vi "符合分析1.7.vi"(5 "大于信号周期":dbl, 6 "length":dbl=200.0 format="%#_13g", 7 "小于信号周期":dbl=500000.0, 8 "min bin":i32=100, 9 "通道B":i32=12, 10 "通道A":i32=1, 11 "file path (dialog if empty)":path=path "G:/tdc/2017/data/test_20250731_124932.csv") -> (0 "standard deviation[ps]":dbl=0.476370061755716 format="%0.2f", 1 "Fitting Sigma":dbl=0.8923286870726619, 2 "Fitting center":dbl=0.5, 3 "mean[ps]":dbl=-0.34797707935405453 format="%0.2f")   [LabVIEW 2017]
uses:
  <vilib>/Utility/file.llb/Read Delimited Spreadsheet (DBL).vi
  <vilib>/Analysis/NI_AALBase.lvlib
panel:
  out "Numeric 2":dbl=110111087360.0 format="%#_16f"
  out "Numeric":dbl=110111087360.0 format="%#_16f"
  out "求和":dbl
  out "x/y":dbl=nan
  out "已经读取的行数":i32=40006
  in  "type (empty)":dbl[][](array[numeric]) caption="类型（空）" format="%0.2f"
  out "错误输出":errorcluster={"status"=TRUE, "code"=4, "source"="Read from Text File in 符合分析1.7.vi<APPEND>\nG:\\tdc\\2017\\data\\test_20250731_124932.csv"}
  in  "单词循环读取的行数":i32=20003
  out "mean[ps] 3":dbl=-185.2719139547909 format="%0.2f"
  out "mean[ps] 2":dbl=-343.16432726517195 format="%0.2f"
  in  "single board":bool=TRUE
  out "offset1":dbl
  out "size(s) 3":i32=64
  in  "calib":bool
  out "offset0":dbl
  in  "file path (dialog if empty) 2":path=path "D:/labview/diff.csv"
  out "数值":i32=2110
  out "大小":i32
  out "Histogram 2":dynamicdata(graph)=[{"t0"=timestamp(500000 s since 1904-01-01), "dt"=1000000.0, "Y"=array[1000 elements], "attributes"=variant("NI_ChannelName"=variant(string " (Histogram)"), "NI_ExpIsRelativeTime"=variant(bool TRUE), "NI_ExpStartTimeStamp"=variant(timestamp timestamp(3836782584.3645935 s since 1904-01-01)), "NI_ExpTimeStamp"=variant(timestamp timestamp(3836782584.3645935 s since 1904-01-01)), "NI_ExpXDimension"=variant(string "BIN"), "NI_OriginalChannelName"=variant(string ""))}] caption="直方图"
  in  "禁用的索引 (列)":i32=6
  in  "window":dbl=200.0 format="%#_13g"
  in  "intervals":i32=1000
  in  "min":dbl=-500.0 format="%#_13g"
  in  "max":dbl=500.0 format="%#_13g"
  out "XY Graph":cluster{"X":dbl, "Y":dbl}[](graph)=[{"X"=107773084761.0, "Y"=0.0}, {"X"=107774084760.0, "Y"=-1.0}, {"X"=107775084760.0, "Y"=0.0}, {"X"=107778084768.0, "Y"=-1.0}, {"X"=107779084768.0, "Y"=0.0}, {"X"=107782084777.0, "Y"=0.0}, {"X"=107793084792.0, "Y"=0.0}, {"X"=107805084816.0, "Y"=-1.0}, {"X"=107809084825.0, "Y"=0.0}, {"X"=107810084824.0, "Y"=-1.0}, {"X"=107814084832.0, "Y"=-1.0}, {"X"=107818084841.0, "Y"=0.0}, {"X"=107827084857.0, "Y"=0.0}, {"X"=107829084856.0, "Y"=0.0}, {"X"=107832084864.0, "Y"=-1.0}, {"X"=107833084864.0, "Y"=0.0}, {"X"=107836084873.0, "Y"=0.0}, {"X"=107837084872.0, "Y"=-1.0}, {"X"=107841084880.0, "Y"=-1.0}, {"X"=107851084896.0, "Y"=0.0}, {"X"=107856084840.0, "Y"=0.0}, {"X"=107859084848.0, "Y"=-1.0}, {"X"=107860084848.0, "Y"=0.0}, {"X"=107863084857.0, "Y"=0.0}, {"X"=107868084864.0, "Y"=-1.0}, {"X"=107872084873.0, "Y"=0.0}, {"X"=107873084872.0, "Y"=-1.0}, {"X"=107878084880.0, "Y"=0.0}, {"X"=107883084888.0, "Y"=0.0}, {"X"=107887084896.0, "Y"=0.0}, {"X"=107891084904.0, "Y"=-1.0}, {"X"=107892084904.0, "Y"=0.0}, {"X"=107895084912.0, "Y"=-1.0}, {"X"=107896084912.0, "Y"=0.0}, {"X"=107899084921.0, "Y"=0.0}, {"X"=107900084920.0, "Y"=-1.0}, {"X"=107901084920.0, "Y"=0.0}, {"X"=107910084904.0, "Y"=0.0}, {"X"=107914084912.0, "Y"=0.0}, {"X"=107915084912.0, "Y"=0.0}, {"X"=107919084920.0, "Y"=0.0}, {"X"=107926084937.0, "Y"=0.0}, {"X"=107935084953.0, "Y"=0.0}, {"X"=107941084960.0, "Y"=0.0}, {"X"=107944084969.0, "Y"=0.0}, {"X"=107950084976.0, "Y"=0.0}, {"X"=107951084976.0, "Y"=0.0}, {"X"=107954084984.0, "Y"=-1.0}, {"X"=107958084993.0, "Y"=0.0}, {"X"=107960084992.0, "Y"=0.0}, {"X"=107963085000.0, "Y"=-1.0}, {"X"=107969085008.0, "Y"=0.0}, {"X"=107973085016.0, "Y"=0.0}, {"X"=107978085024.0, "Y"=0.0}, {"X"=107985085041.0, "Y"=0.0}, {"X"=107994085057.0, "Y"=0.0}, {"X"=108000085064.0, "Y"=0.0}, {"X"=108004085072.0, "Y"=-1.0}, {"X"=108005085072.0, "Y"=0.0}, {"X"=108007085081.0, "Y"=0.0}, {"X"=108008085080.0, "Y"=-1.0}, {"X"=108009085080.0, "Y"=0.0}, {"X"=108012085089.0, "Y"=0.0}, {"X"=108013085088.0, "Y"=-1.0}, {"X"=108014085088.0, "Y"=0.0}, {"X"=108021085105.0, "Y"=0.0}, {"X"=108022085104.0, "Y"=0.0}, {"X"=108023085104.0, "Y"=0.0}, {"X"=108026085112.0, "Y"=-1.0}, {"X"=108027085112.0, "Y"=0.0}, {"X"=108031085120.0, "Y"=-1.0}, {"X"=108032085120.0, "Y"=0.0}, {"X"=108036085128.0, "Y"=0.0}, {"X"=108039085137.0, "Y"=0.0}, {"X"=108041085136.0, "Y"=0.0}, {"X"=108044085144.0, "Y"=-1.0}, {"X"=108048085153.0, "Y"=0.0}, {"X"=108058085168.0, "Y"=-1.0}, {"X"=108059085168.0, "Y"=0.0}, {"X"=108063085176.0, "Y"=0.0}, {"X"=108066085185.0, "Y"=0.0}, {"X"=108067085184.0, "Y"=-1.0}, {"X"=108075085201.0, "Y"=0.0}, {"X"=108080085208.0, "Y"=-1.0}, {"X"=108085085216.0, "Y"=-1.0}, {"X"=108086085216.0, "Y"=0.0}, {"X"=108090085224.0, "Y"=0.0}, {"X"=108094085232.0, "Y"=-1.0}, {"X"=108097085241.0, "Y"=0.0}, {"X"=108116085272.0, "Y"=-1.0}, {"X"=108117085272.0, "Y"=0.0}, {"X"=108121085280.0, "Y"=-1.0}, {"X"=108125085288.0, "Y"=-1.0}, {"X"=108129085297.0, "Y"=0.0}, {"X"=108138085313.0, "Y"=0.0}, {"X"=108143085240.0, "Y"=-1.0}, {"X"=108144085240.0, "Y"=0.0}, {"X"=108148085248.0, "Y"=-1.0}, {"X"=108149085248.0, "Y"=0.0}, {"X"=108153085256.0, "Y"=0.0}, {"X"=108156085265.0, "Y"=0.0}, {"X"=108175085296.0, "Y"=-1.0}, {"X"=108179085304.0, "Y"=-1.0}, {"X"=108187085321.0, "Y"=0.0}, {"X"=108188085320.0, "Y"=-1.0}, {"X"=108197085336.0, "Y"=-1.0}, {"X"=108203085344.0, "Y"=0.0}, {"X"=108207085288.0, "Y"=0.0}, {"X"=108219085313.0, "Y"=0.0}, {"X"=108225085320.0, "Y"=0.0}, {"X"=108233085336.0, "Y"=-1.0}, {"X"=108234085336.0, "Y"=0.0}, {"X"=108238085344.0, "Y"=-1.0}, {"X"=108242085352.0, "Y"=-1.0}, {"X"=108243085352.0, "Y"=0.0}, {"X"=108246085361.0, "Y"=0.0}, {"X"=108247085360.0, "Y"=-1.0}, {"X"=108252085368.0, "Y"=0.0}, {"X"=108256085376.0, "Y"=-1.0}, {"X"=108257085376.0, "Y"=0.0}, {"X"=108261085384.0, "Y"=0.0}, {"X"=108265085392.0, "Y"=-1.0}, {"X"=108266085392.0, "Y"=0.0}, {"X"=108269085400.0, "Y"=-1.0}, {"X"=108273085409.0, "Y"=0.0}, {"X"=108275085408.0, "Y"=0.0}, {"X"=108277085417.0, "Y"=0.0}, {"X"=108284085392.0, "Y"=0.0}, {"X"=108287085400.0, "Y"=-1.0}, {"X"=108292085408.0, "Y"=-1.0}, {"X"=108296085416.0, "Y"=-1.0}, {"X"=108300085425.0, "Y"=0.0}, {"X"=108301085424.0, "Y"=-1.0}, {"X"=108305085432.0, "Y"=-1.0}, {"X"=108306085432.0, "Y"=0.0}, {"X"=108309085441.0, "Y"=0.0}, {"X"=108311085440.0, "Y"=0.0}, {"X"=108314085448.0, "Y"=-1.0}, {"X"=108319085456.0, "Y"=-1.0}, {"X"=108324085464.0, "Y"=0.0}, {"X"=108328085472.0, "Y"=-1.0}, {"X"=108331085481.0, "Y"=0.0}, {"X"=108333085480.0, "Y"=0.0}, {"X"=108336085489.0, "Y"=0.0}, {"X"=108340085497.0, "Y"=0.0}, {"X"=108345085505.0, "Y"=0.0}, {"X"=108350085512.0, "Y"=-1.0}, {"X"=108355085520.0, "Y"=-1.0}, {"X"=108359085528.0, "Y"=-1.0}, {"X"=108367085545.0, "Y"=0.0}, {"X"=108374085552.0, "Y"=0.0}, {"X"=108378085448.0, "Y"=0.0}, {"X"=108386085464.0, "Y"=-1.0}, {"X"=108387085464.0, "Y"=0.0}, {"X"=108390085473.0, "Y"=0.0}, {"X"=108409085504.0, "Y"=-1.0}, {"X"=108417085521.0, "Y"=0.0}, {"X"=108418085520.0, "Y"=0.0}, {"X"=108421085529.0, "Y"=0.0}, {"X"=108436085552.0, "Y"=0.0}, {"X"=108437085552.0, "Y"=0.0}, {"X"=108440085560.0, "Y"=-1.0}, {"X"=108441085560.0, "Y"=0.0}, {"X"=108445085568.0, "Y"=-1.0}, {"X"=108448085577.0, "Y"=0.0}, {"X"=108462085601.0, "Y"=0.0}, {"X"=108464085600.0, "Y"=0.0}, {"X"=108467085608.0, "Y"=-1.0}, {"X"=108468085608.0, "Y"=0.0}, {"X"=108471085617.0, "Y"=0.0}, {"X"=108472085616.0, "Y"=0.0}, {"X"=108475085625.0, "Y"=0.0}, {"X"=108476085624.0, "Y"=-1.0}, {"X"=108480085633.0, "Y"=0.0}, {"X"=108484085641.0, "Y"=0.0}, {"X"=108485085640.0, "Y"=-1.0}, {"X"=108491085648.0, "Y"=0.0}, {"X"=108494085656.0, "Y"=-1.0}, {"X"=108495085656.0, "Y"=0.0}, {"X"=108499085664.0, "Y"=0.0}, {"X"=108500085664.0, "Y"=0.0}, {"X"=108509085680.0, "Y"=0.0}, {"X"=108511085689.0, "Y"=0.0}, {"X"=108518085696.0, "Y"=0.0}, {"X"=108521085704.0, "Y"=-1.0}, {"X"=108530085688.0, "Y"=-1.0}, {"X"=108534085697.0, "Y"=0.0}, {"X"=108538085705.0, "Y"=0.0}, {"X"=108539085704.0, "Y"=-1.0}, {"X"=108543085713.0, "Y"=0.0}, {"X"=108549085720.0, "Y"=0.0}, {"X"=108553085728.0, "Y"=0.0}, {"X"=108554085728.0, "Y"=0.0}, {"X"=108557085736.0, "Y"=-1.0}, {"X"=108558085736.0, "Y"=0.0}, {"X"=108562085744.0, "Y"=0.0}, {"X"=108565085753.0, "Y"=0.0}, {"X"=108581085680.0, "Y"=0.0}, {"X"=108584085688.0, "Y"=-1.0}, {"X"=108592085705.0, "Y"=0.0}, {"X"=108593085704.0, "Y"=-1.0}, {"X"=108597085713.0, "Y"=0.0}, {"X"=108601085721.0, "Y"=0.0}, {"X"=108608085728.0, "Y"=0.0}, {"X"=108612085736.0, "Y"=0.0}, {"X"=108616085744.0, "Y"=0.0}, {"X"=108620085752.0, "Y"=-1.0}, {"X"=108621085752.0, "Y"=0.0}, {"X"=108643085648.0, "Y"=0.0}, {"X"=108647085656.0, "Y"=-1.0}, {"X"=108652085664.0, "Y"=0.0}, {"X"=108655085609.0, "Y"=0.0}, {"X"=108662085616.0, "Y"=0.0}, {"X"=108666085624.0, "Y"=0.0}, {"X"=108670085632.0, "Y"=0.0}, {"X"=108671085632.0, "Y"=0.0}, {"X"=108674085640.0, "Y"=-1.0}, {"X"=108675085640.0, "Y"=0.0}, {"X"=108678085649.0, "Y"=0.0}, {"X"=108680085648.0, "Y"=0.0}, {"X"=108682085657.0, "Y"=0.0}, {"X"=108684085656.0, "Y"=0.0}, {"X"=108689085664.0, "Y"=0.0}, {"X"=108693085672.0, "Y"=0.0}, {"X"=108696085681.0, "Y"=0.0}, {"X"=108698085680.0, "Y"=0.0}, {"X"=108701085688.0, "Y"=-1.0}, {"X"=108705085697.0, "Y"=0.0}, {"X"=108706085696.0, "Y"=0.0}, {"X"=108710085704.0, "Y"=-1.0}, {"X"=108711085704.0, "Y"=0.0}, {"X"=108714085713.0, "Y"=0.0}, {"X"=108716085712.0, "Y"=0.0}, {"X"=108718085721.0, "Y"=0.0}, {"X"=108720085720.0, "Y"=0.0}, {"X"=108725085728.0, "Y"=0.0}, {"X"=108729085736.0, "Y"=0.0}, {"X"=108733085744.0, "Y"=0.0}, {"X"=108737085752.0, "Y"=-1.0}, {"X"=108742085760.0, "Y"=0.0}, {"X"=108752085712.0, "Y"=0.0}, {"X"=108760085728.0, "Y"=-1.0}, {"X"=108764085736.0, "Y"=-1.0}, {"X"=108768085745.0, "Y"=0.0}, {"X"=108769085744.0, "Y"=-1.0}, {"X"=108772085753.0, "Y"=0.0}, {"X"=108773085752.0, "Y"=-1.0}, {"X"=108779085760.0, "Y"=0.0}, {"X"=108783085768.0, "Y"=0.0}, {"X"=108786085777.0, "Y"=0.0}, {"X"=108787085776.0, "Y"=-1.0}, {"X"=108788085776.0, "Y"=0.0}, {"X"=108791085784.0, "Y"=-1.0}, {"X"=108792085784.0, "Y"=0.0}, {"X"=108795085793.0, "Y"=0.0}, {"X"=108796085792.0, "Y"=-1.0}, {"X"=108801085800.0, "Y"=0.0}, {"X"=108815085744.0, "Y"=0.0}, {"X"=108818085752.0, "Y"=-1.0}, {"X"=108822085761.0, "Y"=0.0}, {"X"=108823085760.0, "Y"=-1.0}, {"X"=108827085768.0, "Y"=-1.0}, {"X"=108837085656.0, "Y"=0.0}, {"X"=108842085664.0, "Y"=0.0}, {"X"=108845085672.0, "Y"=-1.0}, {"X"=108854085688.0, "Y"=-1.0}, {"X"=108869085712.0, "Y"=0.0}, {"X"=108873085720.0, "Y"=0.0}, {"X"=108876085729.0, "Y"=0.0}, {"X"=108881085736.0, "Y"=-1.0}, {"X"=108885085745.0, "Y"=0.0}, {"X"=108895085632.0, "Y"=-1.0}, {"X"=108896085632.0, "Y"=0.0}, {"X"=108900085640.0, "Y"=0.0}, {"X"=108904085648.0, "Y"=-1.0}, {"X"=108905085648.0, "Y"=0.0}, {"X"=108908085656.0, "Y"=-1.0}, {"X"=108913085664.0, "Y"=-1.0}, {"X"=108917085672.0, "Y"=-1.0}, {"X"=108923085680.0, "Y"=0.0}, {"X"=108927085688.0, "Y"=0.0}, {"X"=108932085696.0, "Y"=0.0}, {"X"=108935085704.0, "Y"=-1.0}, {"X"=108939085713.0, "Y"=0.0}, {"X"=108944085720.0, "Y"=-1.0}, {"X"=108948085729.0, "Y"=0.0}, {"X"=108954085736.0, "Y"=0.0}, {"X"=108957085745.0, "Y"=0.0}, {"X"=108958085744.0, "Y"=-1.0}, {"X"=108959085744.0, "Y"=0.0}, {"X"=108962085752.0, "Y"=-1.0}, {"X"=108963085752.0, "Y"=0.0}, {"X"=108966085761.0, "Y"=0.0}, {"X"=108967085760.0, "Y"=-1.0}, {"X"=108971085768.0, "Y"=-1.0}, {"X"=108976085776.0, "Y"=-1.0}, {"X"=108981085784.0, "Y"=0.0}, {"X"=108986085792.0, "Y"=0.0}, {"X"=108993085809.0, "Y"=0.0}, {"X"=108994085808.0, "Y"=-1.0}, {"X"=108995085808.0, "Y"=0.0}, {"X"=108998085816.0, "Y"=-1.0}, {"X"=109003085824.0, "Y"=-1.0}, {"X"=109017085848.0, "Y"=0.0}, {"X"=109020085857.0, "Y"=0.0}, {"X"=109021085856.0, "Y"=-1.0}, {"X"=109022085856.0, "Y"=0.0}, {"X"=109025085864.0, "Y"=-1.0}, {"X"=109026085864.0, "Y"=0.0}, {"X"=109029085873.0, "Y"=0.0}, {"X"=109040085888.0, "Y"=0.0}, {"X"=109044085896.0, "Y"=0.0}, {"X"=109045085896.0, "Y"=0.0}, {"X"=109049085904.0, "Y"=0.0}, {"X"=109054085912.0, "Y"=0.0}, {"X"=109056085921.0, "Y"=0.0}, {"X"=109066085936.0, "Y"=-1.0}, {"X"=109071085944.0, "Y"=0.0}, {"X"=109075085952.0, "Y"=-1.0}, {"X"=109076085952.0, "Y"=0.0}, {"X"=109079085960.0, "Y"=-1.0}, {"X"=109083085969.0, "Y"=0.0}, {"X"=109084085968.0, "Y"=-1.0}, {"X"=109088085976.0, "Y"=-1.0}, {"X"=109098085992.0, "Y"=0.0}, {"X"=109099085992.0, "Y"=0.0}, {"X"=109103086000.0, "Y"=0.0}, {"X"=109107086008.0, "Y"=0.0}, {"X"=109110086017.0, "Y"=0.0}, {"X"=109119086033.0, "Y"=0.0}, {"X"=109129086048.0, "Y"=-1.0}, {"X"=109134086056.0, "Y"=0.0}, {"X"=109137086065.0, "Y"=0.0}, {"X"=109138086064.0, "Y"=-1.0}, {"X"=109142086072.0, "Y"=-1.0}, {"X"=109144086072.0, "Y"=0.0}, {"X"=109146086081.0, "Y"=0.0}, {"X"=109147086080.0, "Y"=-1.0}, {"X"=109157086096.0, "Y"=0.0}, {"X"=109161086104.0, "Y"=0.0}, {"X"=109162086104.0, "Y"=0.0}, {"X"=109166086112.0, "Y"=0.0}, {"X"=109169086120.0, "Y"=-1.0}, {"X"=109171086008.0, "Y"=0.0}, {"X"=109173086017.0, "Y"=0.0}, {"X"=109182086033.0, "Y"=0.0}, {"X"=109188086040.0, "Y"=0.0}, {"X"=109192086048.0, "Y"=-1.0}, {"X"=109193086048.0, "Y"=0.0}, {"X"=109196086056.0, "Y"=-1.0}, {"X"=109200086065.0, "Y"=0.0}, {"X"=109205086072.0, "Y"=-1.0}, {"X"=109207086072.0, "Y"=0.0}, {"X"=109210086080.0, "Y"=-1.0}, {"X"=109215086088.0, "Y"=0.0}, {"X"=109216086088.0, "Y"=0.0}, {"X"=109220086096.0, "Y"=0.0}, {"X"=109224086104.0, "Y"=0.0}, {"X"=109225086104.0, "Y"=0.0}, {"X"=109227086113.0, "Y"=0.0}, {"X"=109229086112.0, "Y"=0.0}, {"X"=109232086120.0, "Y"=-1.0}, {"X"=109234086120.0, "Y"=0.0}, {"X"=109241086136.0, "Y"=-1.0}, {"X"=109243086136.0, "Y"=0.0}, {"X"=109246086144.0, "Y"=-1.0}, {"X"=109247086144.0, "Y"=0.0}, {"X"=109251086152.0, "Y"=0.0}, {"X"=109255086160.0, "Y"=-1.0}, {"X"=109256086160.0, "Y"=0.0}, {"X"=109259086168.0, "Y"=-1.0}, {"X"=109263086177.0, "Y"=0.0}, {"X"=109270086184.0, "Y"=0.0}, {"X"=109274086192.0, "Y"=0.0}, {"X"=109278086200.0, "Y"=0.0}, {"X"=109282086208.0, "Y"=-1.0}, {"X"=109283086208.0, "Y"=0.0}, {"X"=109290086225.0, "Y"=0.0}, {"X"=109305086248.0, "Y"=0.0}, {"X"=109309086256.0, "Y"=-1.0}, {"X"=109313086264.0, "Y"=-1.0}, {"X"=109317086273.0, "Y"=0.0}, {"X"=109318086272.0, "Y"=-1.0}, {"X"=109322086280.0, "Y"=-1.0}, {"X"=109328086288.0, "Y"=0.0}, {"X"=109337086304.0, "Y"=0.0}, {"X"=109341086312.0, "Y"=0.0}, {"X"=109344086321.0, "Y"=0.0}, {"X"=109346086320.0, "Y"=0.0}, {"X"=109353086337.0, "Y"=0.0}, {"X"=109358086344.0, "Y"=-1.0}, {"X"=109363086352.0, "Y"=-1.0}, {"X"=109368086360.0, "Y"=0.0}, {"X"=109371086369.0, "Y"=0.0}, {"X"=109372086368.0, "Y"=-1.0}, {"X"=109376086376.0, "Y"=-1.0}, {"X"=109380086385.0, "Y"=0.0}, {"X"=109385086392.0, "Y"=-1.0}, {"X"=109387086392.0, "Y"=0.0}, {"X"=109390086400.0, "Y"=-1.0}, {"X"=109391086400.0, "Y"=0.0}, {"X"=109395086408.0, "Y"=0.0}, {"X"=109400086416.0, "Y"=0.0}, {"X"=109403086424.0, "Y"=-1.0}, {"X"=109405086424.0, "Y"=0.0}, {"X"=109407086433.0, "Y"=0.0}, {"X"=109409086432.0, "Y"=0.0}, {"X"=109416086449.0, "Y"=0.0}, {"X"=109422086456.0, "Y"=0.0}, {"X"=109425086465.0, "Y"=0.0}, {"X"=109426086464.0, "Y"=-1.0}, {"X"=109430086472.0, "Y"=-1.0}, {"X"=109431086472.0, "Y"=0.0}, {"X"=109434086481.0, "Y"=0.0}, {"X"=109439086488.0, "Y"=-1.0}, {"X"=109440086488.0, "Y"=0.0}, {"X"=109441086488.0, "Y"=0.0}, {"X"=109444086496.0, "Y"=-1.0}, {"X"=109449086504.0, "Y"=0.0}, {"X"=109450086504.0, "Y"=0.0}, {"X"=109453086448.0, "Y"=-1.0}, {"X"=109454086448.0, "Y"=0.0}, {"X"=109458086456.0, "Y"=0.0}, {"X"=109459086456.0, "Y"=0.0}, {"X"=109461086465.0, "Y"=0.0}, {"X"=109463086464.0, "Y"=0.0}, {"X"=109468086472.0, "Y"=0.0}, {"X"=109470086481.0, "Y"=0.0}, {"X"=109475086488.0, "Y"=-1.0}, {"X"=109477086488.0, "Y"=0.0}, {"X"=109480086496.0, "Y"=-1.0}, {"X"=109484086504.0, "Y"=-1.0}, {"X"=109485086504.0, "Y"=0.0}, {"X"=109493086520.0, "Y"=-1.0}, {"X"=109497086529.0, "Y"=0.0}, {"X"=109508086544.0, "Y"=0.0}, {"X"=109512086552.0, "Y"=0.0}, {"X"=109524086577.0, "Y"=0.0}, {"X"=109531086584.0, "Y"=0.0}, {"X"=109543086608.0, "Y"=-1.0}, {"X"=109547086616.0, "Y"=-1.0}, {"X"=109551086625.0, "Y"=0.0}, {"X"=109556086632.0, "Y"=-1.0}, {"X"=109558086632.0, "Y"=0.0}, {"X"=109562086640.0, "Y"=0.0}, {"X"=109566086648.0, "Y"=0.0}, {"X"=109567086648.0, "Y"=0.0}, {"X"=109570086656.0, "Y"=-1.0}, {"X"=109571086656.0, "Y"=0.0}, {"X"=109574086664.0, "Y"=-1.0}, {"X"=109575086664.0, "Y"=0.0}, {"X"=109578086673.0, "Y"=0.0}, {"X"=109580086672.0, "Y"=0.0}, {"X"=109585086680.0, "Y"=0.0}, {"X"=109587086689.0, "Y"=0.0}, {"X"=109592086696.0, "Y"=-1.0}, {"X"=109594086696.0, "Y"=0.0}, {"X"=109597086704.0, "Y"=-1.0}, {"X"=109601086712.0, "Y"=-1.0}, {"X"=109602086712.0, "Y"=0.0}, {"X"=109605086721.0, "Y"=0.0}, {"X"=109606086720.0, "Y"=-1.0}, {"X"=109614086737.0, "Y"=0.0}, {"X"=109615086736.0, "Y"=-1.0}, {"X"=109619086744.0, "Y"=-1.0}, {"X"=109621086744.0, "Y"=0.0}, {"X"=109624086752.0, "Y"=-1.0}, {"X"=109625086752.0, "Y"=0.0}, {"X"=109629086760.0, "Y"=0.0}, {"X"=109633086768.0, "Y"=-1.0}, {"X"=109634086768.0, "Y"=0.0}, {"X"=109641086785.0, "Y"=0.0}, {"X"=109643086784.0, "Y"=0.0}, {"X"=109646086792.0, "Y"=-1.0}, {"X"=109648086792.0, "Y"=0.0}, {"X"=109655086808.0, "Y"=-1.0}, {"X"=109656086808.0, "Y"=0.0}, {"X"=109659086817.0, "Y"=0.0}, {"X"=109660086816.0, "Y"=-1.0}, {"X"=109664086825.0, "Y"=0.0}, {"X"=109665086824.0, "Y"=0.0}, {"X"=109668086833.0, "Y"=0.0}, {"X"=109670086832.0, "Y"=0.0}, {"X"=109673086840.0, "Y"=-1.0}, {"X"=109675086840.0, "Y"=0.0}, {"X"=109677086849.0, "Y"=0.0}, {"X"=109679086848.0, "Y"=0.0}, {"X"=109683086856.0, "Y"=0.0}, {"X"=109684086856.0, "Y"=0.0}, {"X"=109687086864.0, "Y"=-1.0}, {"X"=109688086864.0, "Y"=0.0}, {"X"=109692086872.0, "Y"=0.0}, {"X"=109693086872.0, "Y"=0.0}, {"X"=109696086880.0, "Y"=-1.0}, {"X"=109697086880.0, "Y"=0.0}, {"X"=109702086888.0, "Y"=0.0}, {"X"=109711086904.0, "Y"=0.0}, {"X"=109714086912.0, "Y"=-1.0}, {"X"=109718086921.0, "Y"=0.0}, {"X"=109723086928.0, "Y"=-1.0}, {"X"=109733086944.0, "Y"=0.0}, {"X"=109736086953.0, "Y"=0.0}, {"X"=109738086952.0, "Y"=0.0}, {"X"=109742086960.0, "Y"=0.0}, {"X"=109746086968.0, "Y"=0.0}, {"X"=109755086984.0, "Y"=-1.0}, {"X"=109765087000.0, "Y"=0.0}, {"X"=109777087024.0, "Y"=-1.0}, {"X"=109781086953.0, "Y"=0.0}, {"X"=109792086904.0, "Y"=0.0}, {"X"=109796086912.0, "Y"=0.0}, {"X"=109799086921.0, "Y"=0.0}, {"X"=109800086920.0, "Y"=-1.0}, {"X"=109801086920.0, "Y"=0.0}, {"X"=109804086928.0, "Y"=-1.0}, {"X"=109805086928.0, "Y"=0.0}, {"X"=109808086937.0, "Y"=0.0}, {"X"=109809086936.0, "Y"=-1.0}, {"X"=109814086944.0, "Y"=0.0}, {"X"=109819086952.0, "Y"=0.0}, {"X"=109826086969.0, "Y"=0.0}, {"X"=109828086968.0, "Y"=0.0}, {"X"=109831086976.0, "Y"=-1.0}, {"X"=109835086985.0, "Y"=0.0}, {"X"=109836086984.0, "Y"=-1.0}, {"X"=109840086992.0, "Y"=-1.0}, {"X"=109855087016.0, "Y"=0.0}, {"X"=109858087024.0, "Y"=-1.0}, {"X"=109859087024.0, "Y"=0.0}, {"X"=109862087033.0, "Y"=0.0}, {"X"=109863087032.0, "Y"=-1.0}, {"X"=109867087040.0, "Y"=-1.0}, {"X"=109872087048.0, "Y"=-1.0}, {"X"=109877087056.0, "Y"=0.0}, {"X"=109882087064.0, "Y"=0.0}, {"X"=109886087072.0, "Y"=0.0}, {"X"=109889087081.0, "Y"=0.0}, {"X"=109890087080.0, "Y"=-1.0}, {"X"=109894087088.0, "Y"=-1.0}, {"X"=109898087097.0, "Y"=0.0}, {"X"=109899087096.0, "Y"=-1.0}, {"X"=109909087112.0, "Y"=0.0}, {"X"=109913087120.0, "Y"=0.0}, {"X"=109916087129.0, "Y"=0.0}, {"X"=109917087128.0, "Y"=-1.0}, {"X"=109918087128.0, "Y"=0.0}, {"X"=109921087136.0, "Y"=-1.0}, {"X"=109936087080.0, "Y"=0.0}, {"X"=109940087088.0, "Y"=0.0}, {"X"=109945087096.0, "Y"=0.0}, {"X"=109948087104.0, "Y"=-1.0}, {"X"=109952087113.0, "Y"=0.0}, {"X"=109961087129.0, "Y"=0.0}, {"X"=109967087136.0, "Y"=0.0}, {"X"=109971087144.0, "Y"=-1.0}, {"X"=109976087152.0, "Y"=0.0}, {"X"=109979087161.0, "Y"=0.0}, {"X"=109980087160.0, "Y"=-1.0}, {"X"=109984087168.0, "Y"=-1.0}, {"X"=109989087176.0, "Y"=-1.0}, {"X"=109999087192.0, "Y"=0.0}, {"X"=110003087200.0, "Y"=0.0}, {"X"=110006087209.0, "Y"=0.0}, {"X"=110011087216.0, "Y"=-1.0}, {"X"=110020087232.0, "Y"=-1.0}, {"X"=110025087240.0, "Y"=-1.0}, {"X"=110026087240.0, "Y"=0.0}, {"X"=110030087248.0, "Y"=0.0}, {"X"=110033087257.0, "Y"=0.0}, {"X"=110034087256.0, "Y"=-1.0}, {"X"=110035087256.0, "Y"=0.0}, {"X"=110038087264.0, "Y"=-1.0}, {"X"=110042087273.0, "Y"=0.0}, {"X"=110048087280.0, "Y"=0.0}, {"X"=110052087288.0, "Y"=-1.0}, {"X"=110053087288.0, "Y"=0.0}, {"X"=110057087296.0, "Y"=0.0}, {"X"=110061087304.0, "Y"=-1.0}, {"X"=110062087304.0, "Y"=0.0}, {"X"=110065087312.0, "Y"=-1.0}, {"X"=110069087321.0, "Y"=0.0}, {"X"=110070087320.0, "Y"=-1.0}, {"X"=110074087328.0, "Y"=-1.0}, {"X"=110079087304.0, "Y"=-1.0}, {"X"=110084087312.0, "Y"=0.0}, {"X"=110088087320.0, "Y"=-1.0}, {"X"=110089087320.0, "Y"=0.0}, {"X"=110092087328.0, "Y"=-1.0}, {"X"=110093087328.0, "Y"=0.0}, {"X"=110097087336.0, "Y"=-1.0}, {"X"=110101087344.0, "Y"=-1.0}, {"X"=110111087360.0, "Y"=0.0}]
  out "size(s) 2":i32[](array[numeric])=[2111, 128]
  out "Waveform Graph 4":dbl[](graph)
  out "Sum of 3 Gaussians 2":T1(graph)=[{"X Values"=[-29.5, -28.5, -27.5, -26.5, -25.5, -24.5, -23.5, -22.5, -21.5, -20.5, -19.5, -18.5, -17.5, -16.5, -15.5, -14.5, -13.5, -12.5, -11.5, -10.5, -9.5, -8.5, -7.5, -6.5, -5.5, -4.5, -3.5, -2.5, -1.5, -0.5, 0.5, 1.5, 2.5, 3.5, 4.5, 5.5, 6.5, 7.5, 8.5, 9.5, 10.5, 11.5, 12.5, 13.5, 14.5, 15.5, 16.5, 17.5, 18.5, 19.5, 20.5, 21.5, 22.5, 23.5, 24.5, 25.5, 26.5, 27.5, 28.5, 29.5], "Histogram: h(x)"=[1.3602170391502156e-242, 1.6735143296845426e-226, 5.864435467832981e-211, 5.8532697562097335e-196, 1.6639735528091673e-181, 1.3473171896359232e-167, 3.107197321352548e-154, 2.0410017103183032e-141, 3.818505805039623e-129, 2.03478765167168e-117, 3.0883057024660245e-106, 1.3350484442030611e-95, 1.643801295433987e-85, 5.764706003502243e-76, 5.758117995748662e-67, 1.6381720381642473e-58, 1.3274372758385172e-50, 3.063684651472994e-43, 2.013954545794551e-36, 3.7707767427905744e-30, 2.0108863533901428e-24, 3.054356919897459e-19, 1.3213795949910888e-14, 1.6282120264187987e-10, 5.714389934279882e-07, 0.00057122122692905, 0.16263512769810617, 13.188637273370274, 304.621845404808, 2004.0, 3755.0, 2004.0, 304.621845404808, 13.188637273370274, 0.16263512769810617, 0.00057122122692905, 5.714389934279882e-07, 1.6282120264187987e-10, 1.3213795949910888e-14, 3.054356919897459e-19, 2.0108863533901428e-24, 3.7707767427905744e-30, 2.013954545794551e-36, 3.063684651472994e-43, 1.3274372758385172e-50, 1.6381720381642473e-58, 5.758117995748662e-67, 5.764706003502243e-76, 1.643801295433987e-85, 1.3350484442030611e-95, 3.0883057024660245e-106, 2.03478765167168e-117, 3.818505805039623e-129, 2.0410017103183032e-141, 3.107197321352548e-154, 1.3473171896359232e-167, 1.6639735528091673e-181, 5.8532697562097335e-196, 5.864435467832981e-211, 1.6735143296845426e-226]}, {"X Values"=array[1000 elements], "Histogram: h(x)"=array[1000 elements]}]
  out "Fitting center 2":dbl=0.5
  out "Fitting RMS 2":dbl=0.8923286870726619
  in  "min bin 2":i32=30
  in  "length 2":dbl=60.0 format="%#_13g"
  out "Waveform Graph 3":dbl[](graph)
  out "Waveform Graph 2":dbl[](graph)
  out "Sum of 3 Gaussians":T1(graph)=[{"X Values"=[-99.5, -98.5, -97.5, -96.5, -95.5, -94.5, -93.5, -92.5, -91.5, -90.5, -89.5, -88.5, -87.5, -86.5, -85.5, -84.5, -83.5, -82.5, -81.5, -80.5, -79.5, -78.5, -77.5, -76.5, -75.5, -74.5, -73.5, -72.5, -71.5, -70.5, -69.5, -68.5, -67.5, -66.5, -65.5, -64.5, -63.5, -62.5, -61.5, -60.5, -59.5, -58.5, -57.5, -56.5, -55.5, -54.5, -53.5, -52.5, -51.5, -50.5, -49.5, -48.5, -47.5, -46.5, -45.5, -44.5, -43.5, -42.5, -41.5, -40.5, -39.5, -38.5, -37.5, -36.5, -35.5, -34.5, -33.5, -32.5, -31.5, -30.5, -29.5, -28.5, -27.5, -26.5, -25.5, -24.5, -23.5, -22.5, -21.5, -20.5, -19.5, -18.5, -17.5, -16.5, -15.5, -14.5, -13.5, -12.5, -11.5, -10.5, -9.5, -8.5, -7.5, -6.5, -5.5, -4.5, -3.5, -2.5, -1.5, -0.5, 0.5, 1.5, 2.5, 3.5, 4.5, 5.5, 6.5, 7.5, 8.5, 9.5, 10.5, 11.5, 12.5, 13.5, 14.5, 15.5, 16.5, 17.5, 18.5, 19.5, 20.5, 21.5, 22.5, 23.5, 24.5, 25.5, 26.5, 27.5, 28.5, 29.5, 30.5, 31.5, 32.5, 33.5, 34.5, 35.5, 36.5, 37.5, 38.5, 39.5, 40.5, 41.5, 42.5, 43.5, 44.5, 45.5, 46.5, 47.5, 48.5, 49.5, 50.5, 51.5, 52.5, 53.5, 54.5, 55.5, 56.5, 57.5, 58.5, 59.5, 60.5, 61.5, 62.5, 63.5, 64.5, 65.5, 66.5, 67.5, 68.5, 69.5, 70.5, 71.5, 72.5, 73.5, 74.5, 75.5, 76.5, 77.5, 78.5, 79.5, 80.5, 81.5, 82.5, 83.5, 84.5, 85.5, 86.5, 87.5, 88.5, 89.5, 90.5, 91.5, 92.5, 93.5, 94.5, 95.5, 96.5, 97.5, 98.5, 99.5], "Histogram: h(x)"=[0.0, 0.0, 0.0, 0.0, 0.0, 0.0, 0.0, 0.0, 0.0, 0.0, 0.0, 0.0, 0.0, 0.0, 0.0, 0.0, 0.0, 0.0, 0.0, 0.0, 0.0, 0.0, 0.0, 0.0, 0.0, 0.0, 0.0, 0.0, 0.0, 0.0, 0.0, 0.0, 0.0, 0.0, 0.0, 0.0, 0.0, 0.0, 0.0, 0.0, 0.0, 0.0, 0.0, 0.0, 0.0, 0.0, 0.0, 0.0, 0.0, 0.0, 0.0, 0.0, 0.0, 0.0, 0.0, 0.0, 0.0, 0.0, 0.0, 0.0, 0.0, 0.0, 0.0, 0.0, 0.0, 0.0, 2.085829613883e-312, 3.8994005396855046e-294, 2.0763110577758915e-276, 3.148926603343259e-259, 1.3602170391502156e-242, 1.6735143296845426e-226, 5.864435467832981e-211, 5.8532697562097335e-196, 1.6639735528091673e-181, 1.3473171896359232e-167, 3.107197321352548e-154, 2.0410017103183032e-141, 3.818505805039623e-129, 2.03478765167168e-117, 3.0883057024660245e-106, 1.3350484442030611e-95, 1.643801295433987e-85, 5.764706003502243e-76, 5.758117995748662e-67, 1.6381720381642473e-58, 1.3274372758385172e-50, 3.063684651472994e-43, 2.013954545794551e-36, 3.7707767427905744e-30, 2.0108863533901428e-24, 3.054356919897459e-19, 1.3213795949910888e-14, 1.6282120264187987e-10, 5.714389934279882e-07, 0.00057122122692905, 0.16263512769810617, 13.188637273370274, 304.621845404808, 2004.0, 3755.0, 2004.0, 304.621845404808, 13.188637273370274, 0.16263512769810617, 0.00057122122692905, 5.714389934279882e-07, 1.6282120264187987e-10, 1.3213795949910888e-14, 3.054356919897459e-19, 2.0108863533901428e-24, 3.7707767427905744e-30, 2.013954545794551e-36, 3.063684651472994e-43, 1.3274372758385172e-50, 1.6381720381642473e-58, 5.758117995748662e-67, 5.764706003502243e-76, 1.643801295433987e-85, 1.3350484442030611e-95, 3.0883057024660245e-106, 2.03478765167168e-117, 3.818505805039623e-129, 2.0410017103183032e-141, 3.107197321352548e-154, 1.3473171896359232e-167, 1.6639735528091673e-181, 5.8532697562097335e-196, 5.864435467832981e-211, 1.6735143296845426e-226, 1.3602170391502156e-242, 3.148926603343259e-259, 2.0763110577758915e-276, 3.8994005396855046e-294, 2.085829613883e-312, 0.0, 0.0, 0.0, 0.0, 0.0, 0.0, 0.0, 0.0, 0.0, 0.0, 0.0, 0.0, 0.0, 0.0, 0.0, 0.0, 0.0, 0.0, 0.0, 0.0, 0.0, 0.0, 0.0, 0.0, 0.0, 0.0, 0.0, 0.0, 0.0, 0.0, 0.0, 0.0, 0.0, 0.0, 0.0, 0.0, 0.0, 0.0, 0.0, 0.0, 0.0, 0.0, 0.0, 0.0, 0.0, 0.0, 0.0, 0.0, 0.0, 0.0, 0.0, 0.0, 0.0, 0.0, 0.0, 0.0, 0.0, 0.0, 0.0, 0.0, 0.0, 0.0, 0.0, 0.0, 0.0]}, {"X Values"=[-499.5, -498.5, -497.5, -496.5, -495.5, -494.5, -493.5, -492.5, -491.5, -490.5, -489.5, -488.5, -487.5, -486.5, -485.5, -484.5, -483.5, -482.5, -481.5, -480.5, -479.5, -478.5, -477.5, -476.5, -475.5, -474.5, -473.5, -472.5, -471.5, -470.5, -469.5, -468.5, -467.5, -466.5, -465.5, -464.5, -463.5, -462.5, -461.5, -460.5, -459.5, -458.5, -457.5, -456.5, -455.5, -454.5, -453.5, -452.5, -451.5, -450.5, -449.5, -448.5, -447.5, -446.5, -445.5, -444.5, -443.5, -442.5, -441.5, -440.5, -439.5, -438.5, -437.5, -436.5, -435.5, -434.5, -433.5, -432.5, -431.5, -430.5, -429.5, -428.5, -427.5, -426.5, -425.5, -424.5, -423.5, -422.5, -421.5, -420.5, -419.5, -418.5, -417.5, -416.5, -415.5, -414.5, -413.5, -412.5, -411.5, -410.5, -409.5, -408.5, -407.5, -406.5, -405.5, -404.5, -403.5, -402.5, -401.5, -400.5, -399.5, -398.5, -397.5, -396.5, -395.5, -394.5, -393.5, -392.5, -391.5, -390.5, -389.5, -388.5, -387.5, -386.5, -385.5, -384.5, -383.5, -382.5, -381.5, -380.5, -379.5, -378.5, -377.5, -376.5, -375.5, -374.5, -373.5, -372.5, -371.5, -370.5, -369.5, -368.5, -367.5, -366.5, -365.5, -364.5, -363.5, -362.5, -361.5, -360.5, -359.5, -358.5, -357.5, -356.5, -355.5, -354.5, -353.5, -352.5, -351.5, -350.5, -349.5, -348.5, -347.5, -346.5, -345.5, -344.5, -343.5, -342.5, -341.5, -340.5, -339.5, -338.5, -337.5, -336.5, -335.5, -334.5, -333.5, -332.5, -331.5, -330.5, -329.5, -328.5, -327.5, -326.5, -325.5, -324.5, -323.5, -322.5, -321.5, -320.5, -319.5, -318.5, -317.5, -316.5, -315.5, -314.5, -313.5, -312.5, -311.5, -310.5, -309.5, -308.5, -307.5, -306.5, -305.5, -304.5, -303.5, -302.5, -301.5, -300.5, -299.5, -298.5, -297.5, -296.5, -295.5, -294.5, -293.5, -292.5, -291.5, -290.5, -289.5, -288.5, -287.5, -286.5, -285.5, -284.5, -283.5, -282.5, -281.5, -280.5, -279.5, -278.5, -277.5, -276.5, -275.5, -274.5, -273.5, -272.5, -271.5, -270.5, -269.5, -268.5, -267.5, -266.5, -265.5, -264.5, -263.5, -262.5, -261.5, -260.5, -259.5, -258.5, -257.5, -256.5, -255.5, -254.5, -253.5, -252.5, -251.5, -250.5, -249.5, -248.5, -247.5, -246.5, -245.5, -244.5, -243.5, -242.5, -241.5, -240.5, -239.5, -238.5, -237.5, -236.5, -235.5, -234.5, -233.5, -232.5, -231.5, -230.5, -229.5, -228.5, -227.5, -226.5, -225.5, -224.5, -223.5, -222.5, -221.5, -220.5, -219.5, -218.5, -217.5, -216.5, -215.5, -214.5, -213.5, -212.5, -211.5, -210.5, -209.5, -208.5, -207.5, -206.5, -205.5, -204.5, -203.5, -202.5, -201.5, -200.5, -199.5, -198.5, -197.5, -196.5, -195.5, -194.5, -193.5, -192.5, -191.5, -190.5, -189.5, -188.5, -187.5, -186.5, -185.5, -184.5, -183.5, -182.5, -181.5, -180.5, -179.5, -178.5, -177.5, -176.5, -175.5, -174.5, -173.5, -172.5, -171.5, -170.5, -169.5, -168.5, -167.5, -166.5, -165.5, -164.5, -163.5, -162.5, -161.5, -160.5, -159.5, -158.5, -157.5, -156.5, -155.5, -154.5, -153.5, -152.5, -151.5, -150.5, -149.5, -148.5, -147.5, -146.5, -145.5, -144.5, -143.5, -142.5, -141.5, -140.5, -139.5, -138.5, -137.5, -136.5, -135.5, -134.5, -133.5, -132.5, -131.5, -130.5, -129.5, -128.5, -127.5, -126.5, -125.5, -124.5, -123.5, -122.5, -121.5, -120.5, -119.5, -118.5, -117.5, -116.5, -115.5, -114.5, -113.5, -112.5, -111.5, -110.5, -109.5, -108.5, -107.5, -106.5, -105.5, -104.5, -103.5, -102.5, -101.5, -100.5, -99.5, -98.5, -97.5, -96.5, -95.5, -94.5, -93.5, -92.5, -91.5, -90.5, -89.5, -88.5, -87.5, -86.5, -85.5, -84.5, -83.5, -82.5, -81.5, -80.5, -79.5, -78.5, -77.5, -76.5, -75.5, -74.5, -73.5, -72.5, -71.5, -70.5, -69.5, -68.5, -67.5, -66.5, -65.5, -64.5, -63.5, -62.5, -61.5, -60.5, -59.5, -58.5, -57.5, -56.5, -55.5, -54.5, -53.5, -52.5, -51.5, -50.5, -49.5, -48.5, -47.5, -46.5, -45.5, -44.5, -43.5, -42.5, -41.5, -40.5, -39.5, -38.5, -37.5, -36.5, -35.5, -34.5, -33.5, -32.5, -31.5, -30.5, -29.5, -28.5, -27.5, -26.5, -25.5, -24.5, -23.5, -22.5, -21.5, -20.5, -19.5, -18.5, -17.5, -16.5, -15.5, -14.5, -13.5, -12.5, -11.5, -10.5, -9.5, -8.5, -7.5, -6.5, -5.5, -4.5, -3.5, -2.5, -1.5, -0.5, 0.5, 1.5, 2.5, 3.5, 4.5, 5.5, 6.5, 7.5, 8.5, 9.5, 10.5, 11.5, 12.5, 13.5, 14.5, 15.5, 16.5, 17.5, 18.5, 19.5, 20.5, 21.5, 22.5, 23.5, 24.5, 25.5, 26.5, 27.5, 28.5, 29.5, 30.5, 31.5, 32.5, 33.5, 34.5, 35.5, 36.5, 37.5, 38.5, 39.5, 40.5, 41.5, 42.5, 43.5, 44.5, 45.5, 46.5, 47.5, 48.5, 49.5, 50.5, 51.5, 52.5, 53.5, 54.5, 55.5, 56.5, 57.5, 58.5, 59.5, 60.5, 61.5, 62.5, 63.5, 64.5, 65.5, 66.5, 67.5, 68.5, 69.5, 70.5, 71.5, 72.5, 73.5, 74.5, 75.5, 76.5, 77.5, 78.5, 79.5, 80.5, 81.5, 82.5, 83.5, 84.5, 85.5, 86.5, 87.5, 88.5, 89.5, 90.5, 91.5, 92.5, 93.5, 94.5, 95.5, 96.5, 97.5, 98.5, 99.5, 100.5, 101.5, 102.5, 103.5, 104.5, 105.5, 106.5, 107.5, 108.5, 109.5, 110.5, 111.5, 112.5, 113.5, 114.5, 115.5, 116.5, 117.5, 118.5, 119.5, 120.5, 121.5, 122.5, 123.5, 124.5, 125.5, 126.5, 127.5, 128.5, 129.5, 130.5, 131.5, 132.5, 133.5, 134.5, 135.5, 136.5, 137.5, 138.5, 139.5, 140.5, 141.5, 142.5, 143.5, 144.5, 145.5, 146.5, 147.5, 148.5, 149.5, 150.5, 151.5, 152.5, 153.5, 154.5, 155.5, 156.5, 157.5, 158.5, 159.5, 160.5, 161.5, 162.5, 163.5, 164.5, 165.5, 166.5, 167.5, 168.5, 169.5, 170.5, 171.5, 172.5, 173.5, 174.5, 175.5, 176.5, 177.5, 178.5, 179.5, 180.5, 181.5, 182.5, 183.5, 184.5, 185.5, 186.5, 187.5, 188.5, 189.5, 190.5, 191.5, 192.5, 193.5, 194.5, 195.5, 196.5, 197.5, 198.5, 199.5, 200.5, 201.5, 202.5, 203.5, 204.5, 205.5, 206.5, 207.5, 208.5, 209.5, 210.5, 211.5, 212.5, 213.5, 214.5, 215.5, 216.5, 217.5, 218.5, 219.5, 220.5, 221.5, 222.5, 223.5, 224.5, 225.5, 226.5, 227.5, 228.5, 229.5, 230.5, 231.5, 232.5, 233.5, 234.5, 235.5, 236.5, 237.5, 238.5, 239.5, 240.5, 241.5, 242.5, 243.5, 244.5, 245.5, 246.5, 247.5, 248.5, 249.5, 250.5, 251.5, 252.5, 253.5, 254.5, 255.5, 256.5, 257.5, 258.5, 259.5, 260.5, 261.5, 262.5, 263.5, 264.5, 265.5, 266.5, 267.5, 268.5, 269.5, 270.5, 271.5, 272.5, 273.5, 274.5, 275.5, 276.5, 277.5, 278.5, 279.5, 280.5, 281.5, 282.5, 283.5, 284.5, 285.5, 286.5, 287.5, 288.5, 289.5, 290.5, 291.5, 292.5, 293.5, 294.5, 295.5, 296.5, 297.5, 298.5, 299.5, 300.5, 301.5, 302.5, 303.5, 304.5, 305.5, 306.5, 307.5, 308.5, 309.5, 310.5, 311.5, 312.5, 313.5, 314.5, 315.5, 316.5, 317.5, 318.5, 319.5, 320.5, 321.5, 322.5, 323.5, 324.5, 325.5, 326.5, 327.5, 328.5, 329.5, 330.5, 331.5, 332.5, 333.5, 334.5, 335.5, 336.5, 337.5, 338.5, 339.5, 340.5, 341.5, 342.5, 343.5, 344.5, 345.5, 346.5, 347.5, 348.5, 349.5, 350.5, 351.5, 352.5, 353.5, 354.5, 355.5, 356.5, 357.5, 358.5, 359.5, 360.5, 361.5, 362.5, 363.5, 364.5, 365.5, 366.5, 367.5, 368.5, 369.5, 370.5, 371.5, 372.5, 373.5, 374.5, 375.5, 376.5, 377.5, 378.5, 379.5, 380.5, 381.5, 382.5, 383.5, 384.5, 385.5, 386.5, 387.5, 388.5, 389.5, 390.5, 391.5, 392.5, 393.5, 394.5, 395.5, 396.5, 397.5, 398.5, 399.5, 400.5, 401.5, 402.5, 403.5, 404.5, 405.5, 406.5, 407.5, 408.5, 409.5, 410.5, 411.5, 412.5, 413.5, 414.5, 415.5, 416.5, 417.5, 418.5, 419.5, 420.5, 421.5, 422.5, 423.5, 424.5, 425.5, 426.5, 427.5, 428.5, 429.5, 430.5, 431.5, 432.5, 433.5, 434.5, 435.5, 436.5, 437.5, 438.5, 439.5, 440.5, 441.5, 442.5, 443.5, 444.5, 445.5, 446.5, 447.5, 448.5, 449.5, 450.5, 451.5, 452.5, 453.5, 454.5, 455.5, 456.5, 457.5, 458.5, 459.5, 460.5, 461.5, 462.5, 463.5, 464.5, 465.5, 466.5, 467.5, 468.5, 469.5, 470.5, 471.5, 472.5, 473.5, 474.5, 475.5, 476.5, 477.5, 478.5, 479.5, 480.5, 481.5, 482.5, 483.5, 484.5, 485.5, 486.5, 487.5, 488.5, 489.5, 490.5, 491.5, 492.5, 493.5, 494.5, 495.5, 496.5, 497.5, 498.5, 499.5], "Histogram: h(x)"=[0.0, 0.0, 0.0, 0.0, 0.0, 0.0, 0.0, 0.0, 0.0, 0.0, 0.0, 0.0, 0.0, 0.0, 0.0, 0.0, 0.0, 0.0, 0.0, 0.0, 0.0, 0.0, 0.0, 0.0, 0.0, 0.0, 0.0, 0.0, 0.0, 0.0, 0.0, 0.0, 0.0, 0.0, 0.0, 0.0, 0.0, 0.0, 0.0, 0.0, 0.0, 0.0, 0.0, 0.0, 0.0, 0.0, 0.0, 0.0, 0.0, 0.0, 0.0, 0.0, 0.0, 0.0, 0.0, 0.0, 0.0, 0.0, 0.0, 0.0, 0.0, 0.0, 0.0, 0.0, 0.0, 0.0, 0.0, 0.0, 0.0, 0.0, 0.0, 0.0, 0.0, 0.0, 0.0, 0.0, 0.0, 0.0, 0.0, 0.0, 0.0, 0.0, 0.0, 0.0, 0.0, 0.0, 0.0, 0.0, 0.0, 0.0, 0.0, 0.0, 0.0, 0.0, 0.0, 0.0, 0.0, 0.0, 0.0, 0.0, 0.0, 0.0, 0.0, 0.0, 0.0, 0.0, 0.0, 0.0, 0.0, 0.0, 0.0, 0.0, 0.0, 0.0, 0.0, 0.0, 0.0, 0.0, 0.0, 0.0, 0.0, 0.0, 0.0, 0.0, 0.0, 0.0, 0.0, 0.0, 0.0, 0.0, 0.0, 0.0, 0.0, 0.0, 0.0, 0.0, 0.0, 0.0, 0.0, 0.0, 0.0, 0.0, 0.0, 0.0, 0.0, 0.0, 0.0, 0.0, 0.0, 0.0, 0.0, 0.0, 0.0, 0.0, 0.0, 0.0, 0.0, 0.0, 0.0, 0.0, 0.0, 0.0, 0.0, 0.0, 0.0, 0.0, 0.0, 0.0, 0.0, 0.0, 0.0, 0.0, 0.0, 0.0, 0.0, 0.0, 0.0, 0.0, 0.0, 0.0, 0.0, 0.0, 0.0, 0.0, 0.0, 0.0, 0.0, 0.0, 0.0, 0.0, 0.0, 0.0, 0.0, 0.0, 0.0, 0.0, 0.0, 0.0, 0.0, 0.0, 0.0, 0.0, 0.0, 0.0, 0.0, 0.0, 0.0, 0.0, 0.0, 0.0, 0.0, 0.0, 0.0, 0.0, 0.0, 0.0, 0.0, 0.0, 0.0, 0.0, 0.0, 0.0, 0.0, 0.0, 0.0, 0.0, 0.0, 0.0, 0.0, 0.0, 0.0, 0.0, 0.0, 0.0, 0.0, 0.0, 0.0, 0.0, 0.0, 0.0, 0.0, 0.0, 0.0, 0.0, 0.0, 0.0, 0.0, 0.0, 0.0, 0.0, 0.0, 0.0, 0.0, 0.0, 0.0, 0.0, 0.0, 0.0, 0.0, 0.0, 0.0, 0.0, 0.0, 0.0, 0.0, 0.0, 0.0, 0.0, 0.0, 0.0, 0.0, 0.0, 0.0, 0.0, 0.0, 0.0, 0.0, 0.0, 0.0, 0.0, 0.0, 0.0, 0.0, 0.0, 0.0, 0.0, 0.0, 0.0, 0.0, 0.0, 0.0, 0.0, 0.0, 0.0, 0.0, 0.0, 0.0, 0.0, 0.0, 0.0, 0.0, 0.0, 0.0, 0.0, 0.0, 0.0, 0.0, 0.0, 0.0, 0.0, 0.0, 0.0, 0.0, 0.0, 0.0, 0.0, 0.0, 0.0, 0.0, 0.0, 0.0, 0.0, 0.0, 0.0, 0.0, 0.0, 0.0, 0.0, 0.0, 0.0, 0.0, 0.0, 0.0, 0.0, 0.0, 0.0, 0.0, 0.0, 0.0, 0.0, 0.0, 0.0, 0.0, 0.0, 0.0, 0.0, 0.0, 0.0, 0.0, 0.0, 0.0, 0.0, 0.0, 0.0, 0.0, 0.0, 0.0, 0.0, 0.0, 0.0, 0.0, 0.0, 0.0, 0.0, 0.0, 0.0, 0.0, 0.0, 0.0, 0.0, 0.0, 0.0, 0.0, 0.0, 0.0, 0.0, 0.0, 0.0, 0.0, 0.0, 0.0, 0.0, 0.0, 0.0, 0.0, 0.0, 0.0, 0.0, 0.0, 0.0, 0.0, 0.0, 0.0, 0.0, 0.0, 0.0, 0.0, 0.0, 0.0, 0.0, 0.0, 0.0, 0.0, 0.0, 0.0, 0.0, 0.0, 0.0, 0.0, 0.0, 0.0, 0.0, 0.0, 0.0, 0.0, 0.0, 0.0, 0.0, 0.0, 0.0, 0.0, 0.0, 0.0, 0.0, 0.0, 0.0, 0.0, 0.0, 0.0, 0.0, 0.0, 0.0, 0.0, 0.0, 0.0, 0.0, 0.0, 0.0, 0.0, 0.0, 0.0, 0.0, 0.0, 0.0, 0.0, 0.0, 0.0, 0.0, 0.0, 0.0, 0.0, 0.0, 0.0, 0.0, 0.0, 0.0, 0.0, 0.0, 0.0, 0.0, 0.0, 0.0, 0.0, 0.0, 0.0, 0.0, 0.0, 0.0, 0.0, 0.0, 0.0, 0.0, 0.0, 0.0, 0.0, 0.0, 0.0, 0.0, 0.0, 0.0, 0.0, 0.0, 0.0, 0.0, 0.0, 0.0, 0.0, 0.0, 0.0, 0.0, 0.0, 0.0, 0.0, 0.0, 0.0, 0.0, 0.0, 0.0, 0.0, 2004.0, 3755.0, 0.0, 0.0, 0.0, 0.0, 0.0, 0.0, 0.0, 0.0, 0.0, 0.0, 0.0, 0.0, 0.0, 0.0, 0.0, 0.0, 0.0, 0.0, 0.0, 0.0, 0.0, 0.0, 0.0, 0.0, 0.0, 0.0, 0.0, 0.0, 0.0, 0.0, 0.0, 0.0, 0.0, 0.0, 0.0, 0.0, 0.0, 0.0, 0.0, 0.0, 0.0, 0.0, 0.0, 0.0, 0.0, 0.0, 0.0, 0.0, 0.0, 0.0, 0.0, 0.0, 0.0, 0.0, 0.0, 0.0, 0.0, 0.0, 0.0, 0.0, 0.0, 0.0, 0.0, 0.0, 0.0, 0.0, 0.0, 0.0, 0.0, 0.0, 0.0, 0.0, 0.0, 0.0, 0.0, 0.0, 0.0, 0.0, 0.0, 0.0, 0.0, 0.0, 0.0, 0.0, 0.0, 0.0, 0.0, 0.0, 0.0, 0.0, 0.0, 0.0, 0.0, 0.0, 0.0, 0.0, 0.0, 0.0, 0.0, 0.0, 0.0, 0.0, 0.0, 0.0, 0.0, 0.0, 0.0, 0.0, 0.0, 0.0, 0.0, 0.0, 0.0, 0.0, 0.0, 0.0, 0.0, 0.0, 0.0, 0.0, 0.0, 0.0, 0.0, 0.0, 0.0, 0.0, 0.0, 0.0, 0.0, 0.0, 0.0, 0.0, 0.0, 0.0, 0.0, 0.0, 0.0, 0.0, 0.0, 0.0, 0.0, 0.0, 0.0, 0.0, 0.0, 0.0, 0.0, 0.0, 0.0, 0.0, 0.0, 0.0, 0.0, 0.0, 0.0, 0.0, 0.0, 0.0, 0.0, 0.0, 0.0, 0.0, 0.0, 0.0, 0.0, 0.0, 0.0, 0.0, 0.0, 0.0, 0.0, 0.0, 0.0, 0.0, 0.0, 0.0, 0.0, 0.0, 0.0, 0.0, 0.0, 0.0, 0.0, 0.0, 0.0, 0.0, 0.0, 0.0, 0.0, 0.0, 0.0, 0.0, 0.0, 0.0, 0.0, 0.0, 0.0, 0.0, 0.0, 0.0, 0.0, 0.0, 0.0, 0.0, 0.0, 0.0, 0.0, 0.0, 0.0, 0.0, 0.0, 0.0, 0.0, 0.0, 0.0, 0.0, 0.0, 0.0, 0.0, 0.0, 0.0, 0.0, 0.0, 0.0, 0.0, 0.0, 0.0, 0.0, 0.0, 0.0, 0.0, 0.0, 0.0, 0.0, 0.0, 0.0, 0.0, 0.0, 0.0, 0.0, 0.0, 0.0, 0.0, 0.0, 0.0, 0.0, 0.0, 0.0, 0.0, 0.0, 0.0, 0.0, 0.0, 0.0, 0.0, 0.0, 0.0, 0.0, 0.0, 0.0, 0.0, 0.0, 0.0, 0.0, 0.0, 0.0, 0.0, 0.0, 0.0, 0.0, 0.0, 0.0, 0.0, 0.0, 0.0, 0.0, 0.0, 0.0, 0.0, 0.0, 0.0, 0.0, 0.0, 0.0, 0.0, 0.0, 0.0, 0.0, 0.0, 0.0, 0.0, 0.0, 0.0, 0.0, 0.0, 0.0, 0.0, 0.0, 0.0, 0.0, 0.0, 0.0, 0.0, 0.0, 0.0, 0.0, 0.0, 0.0, 0.0, 0.0, 0.0, 0.0, 0.0, 0.0, 0.0, 0.0, 0.0, 0.0, 0.0, 0.0, 0.0, 0.0, 0.0, 0.0, 0.0, 0.0, 0.0, 0.0, 0.0, 0.0, 0.0, 0.0, 0.0, 0.0, 0.0, 0.0, 0.0, 0.0, 0.0, 0.0, 0.0, 0.0, 0.0, 0.0, 0.0, 0.0, 0.0, 0.0, 0.0, 0.0, 0.0, 0.0, 0.0, 0.0, 0.0, 0.0, 0.0, 0.0, 0.0, 0.0, 0.0, 0.0, 0.0, 0.0, 0.0, 0.0, 0.0, 0.0, 0.0, 0.0, 0.0, 0.0, 0.0, 0.0, 0.0, 0.0, 0.0, 0.0, 0.0, 0.0, 0.0, 0.0, 0.0, 0.0, 0.0, 0.0, 0.0, 0.0, 0.0, 0.0, 0.0, 0.0, 0.0, 0.0, 0.0, 0.0, 0.0, 0.0, 0.0, 0.0, 0.0, 0.0, 0.0, 0.0, 0.0, 0.0, 0.0, 0.0, 0.0, 0.0, 0.0, 0.0, 0.0, 0.0, 0.0, 0.0, 0.0, 0.0, 0.0, 0.0, 0.0, 0.0, 0.0, 0.0, 0.0, 0.0, 0.0, 0.0, 0.0, 0.0, 0.0, 0.0, 0.0, 0.0, 0.0, 0.0, 0.0, 0.0, 0.0, 0.0, 0.0, 0.0, 0.0, 0.0, 0.0, 0.0, 0.0, 0.0, 0.0, 0.0, 0.0, 0.0, 0.0, 0.0, 0.0, 0.0, 0.0, 0.0, 0.0, 0.0, 0.0, 0.0, 0.0, 0.0, 0.0, 0.0, 0.0, 0.0, 0.0, 0.0, 0.0, 0.0, 0.0, 0.0, 0.0, 0.0, 0.0, 0.0, 0.0, 0.0, 0.0, 0.0, 0.0, 0.0, 0.0, 0.0, 0.0, 0.0, 0.0, 0.0, 0.0, 0.0, 0.0, 0.0, 0.0, 0.0, 0.0, 0.0, 0.0]}]
  out "Waveform Graph":dbl[](graph)
  in  "time offset":dbl=-320.23
  out "有效符合数":i32=5759
  out "Histogram":dynamicdata(graph)=[{"t0"=timestamp(-49.75 s since 1904-01-01), "dt"=0.5, "Y"=[0.0, 0.0, 0.0, 0.0, 0.0, 0.0, 0.0, 0.0, 0.0, 0.0, 0.0, 0.0, 0.0, 0.0, 0.0, 0.0, 0.0, 0.0, 0.0, 0.0, 0.0, 0.0, 0.0, 0.0, 0.0, 0.0, 0.0, 0.0, 0.0, 0.0, 0.0, 0.0, 0.0, 0.0, 0.0, 0.0, 0.0, 0.0, 0.0, 0.0, 0.0, 0.0, 0.0, 0.0, 0.0, 0.0, 0.0, 0.0, 0.0, 0.0, 0.0, 0.0, 0.0, 0.0, 0.0, 0.0, 0.0, 0.0, 0.0, 0.0, 0.0, 0.0, 0.0, 0.0, 0.0, 0.0, 0.0, 0.0, 0.0, 0.0, 0.0, 0.0, 0.0, 0.0, 0.0, 0.0, 0.0, 0.0, 0.0, 0.0, 0.0, 0.0, 0.0, 0.0, 0.0, 0.0, 0.0, 0.0, 0.0, 0.0, 0.0, 0.0, 0.0, 0.0, 0.0, 0.0, 0.0, 0.0, 2004.0, 0.0, 3755.0, 0.0, 0.0, 0.0, 0.0, 0.0, 0.0, 0.0, 0.0, 0.0, 0.0, 0.0, 0.0, 0.0, 0.0, 0.0, 0.0, 0.0, 0.0, 0.0, 0.0, 0.0, 0.0, 0.0, 0.0, 0.0, 0.0, 0.0, 0.0, 0.0, 0.0, 0.0, 0.0, 0.0, 0.0, 0.0, 0.0, 0.0, 0.0, 0.0, 0.0, 0.0, 0.0, 0.0, 0.0, 0.0, 0.0, 0.0, 0.0, 0.0, 0.0, 0.0, 0.0, 0.0, 0.0, 0.0, 0.0, 0.0, 0.0, 0.0, 0.0, 0.0, 0.0, 0.0, 0.0, 0.0, 0.0, 0.0, 0.0, 0.0, 0.0, 0.0, 0.0, 0.0, 0.0, 0.0, 0.0, 0.0, 0.0, 0.0, 0.0, 0.0, 0.0, 0.0, 0.0, 0.0, 0.0, 0.0, 0.0, 0.0, 0.0, 0.0, 0.0, 0.0, 0.0, 0.0, 0.0, 0.0, 0.0, 0.0], "attributes"=variant("NI_ChannelName"=variant(string " (Histogram)"), "NI_ExpIsRelativeTime"=variant(bool TRUE), "NI_ExpStartTimeStamp"=variant(timestamp timestamp(3836782584.3645935 s since 1904-01-01)), "NI_ExpTimeStamp"=variant(timestamp timestamp(3836782584.3645935 s since 1904-01-01)), "NI_ExpXDimension"=variant(string "BIN"), "NI_OriginalChannelName"=variant(string ""))}]
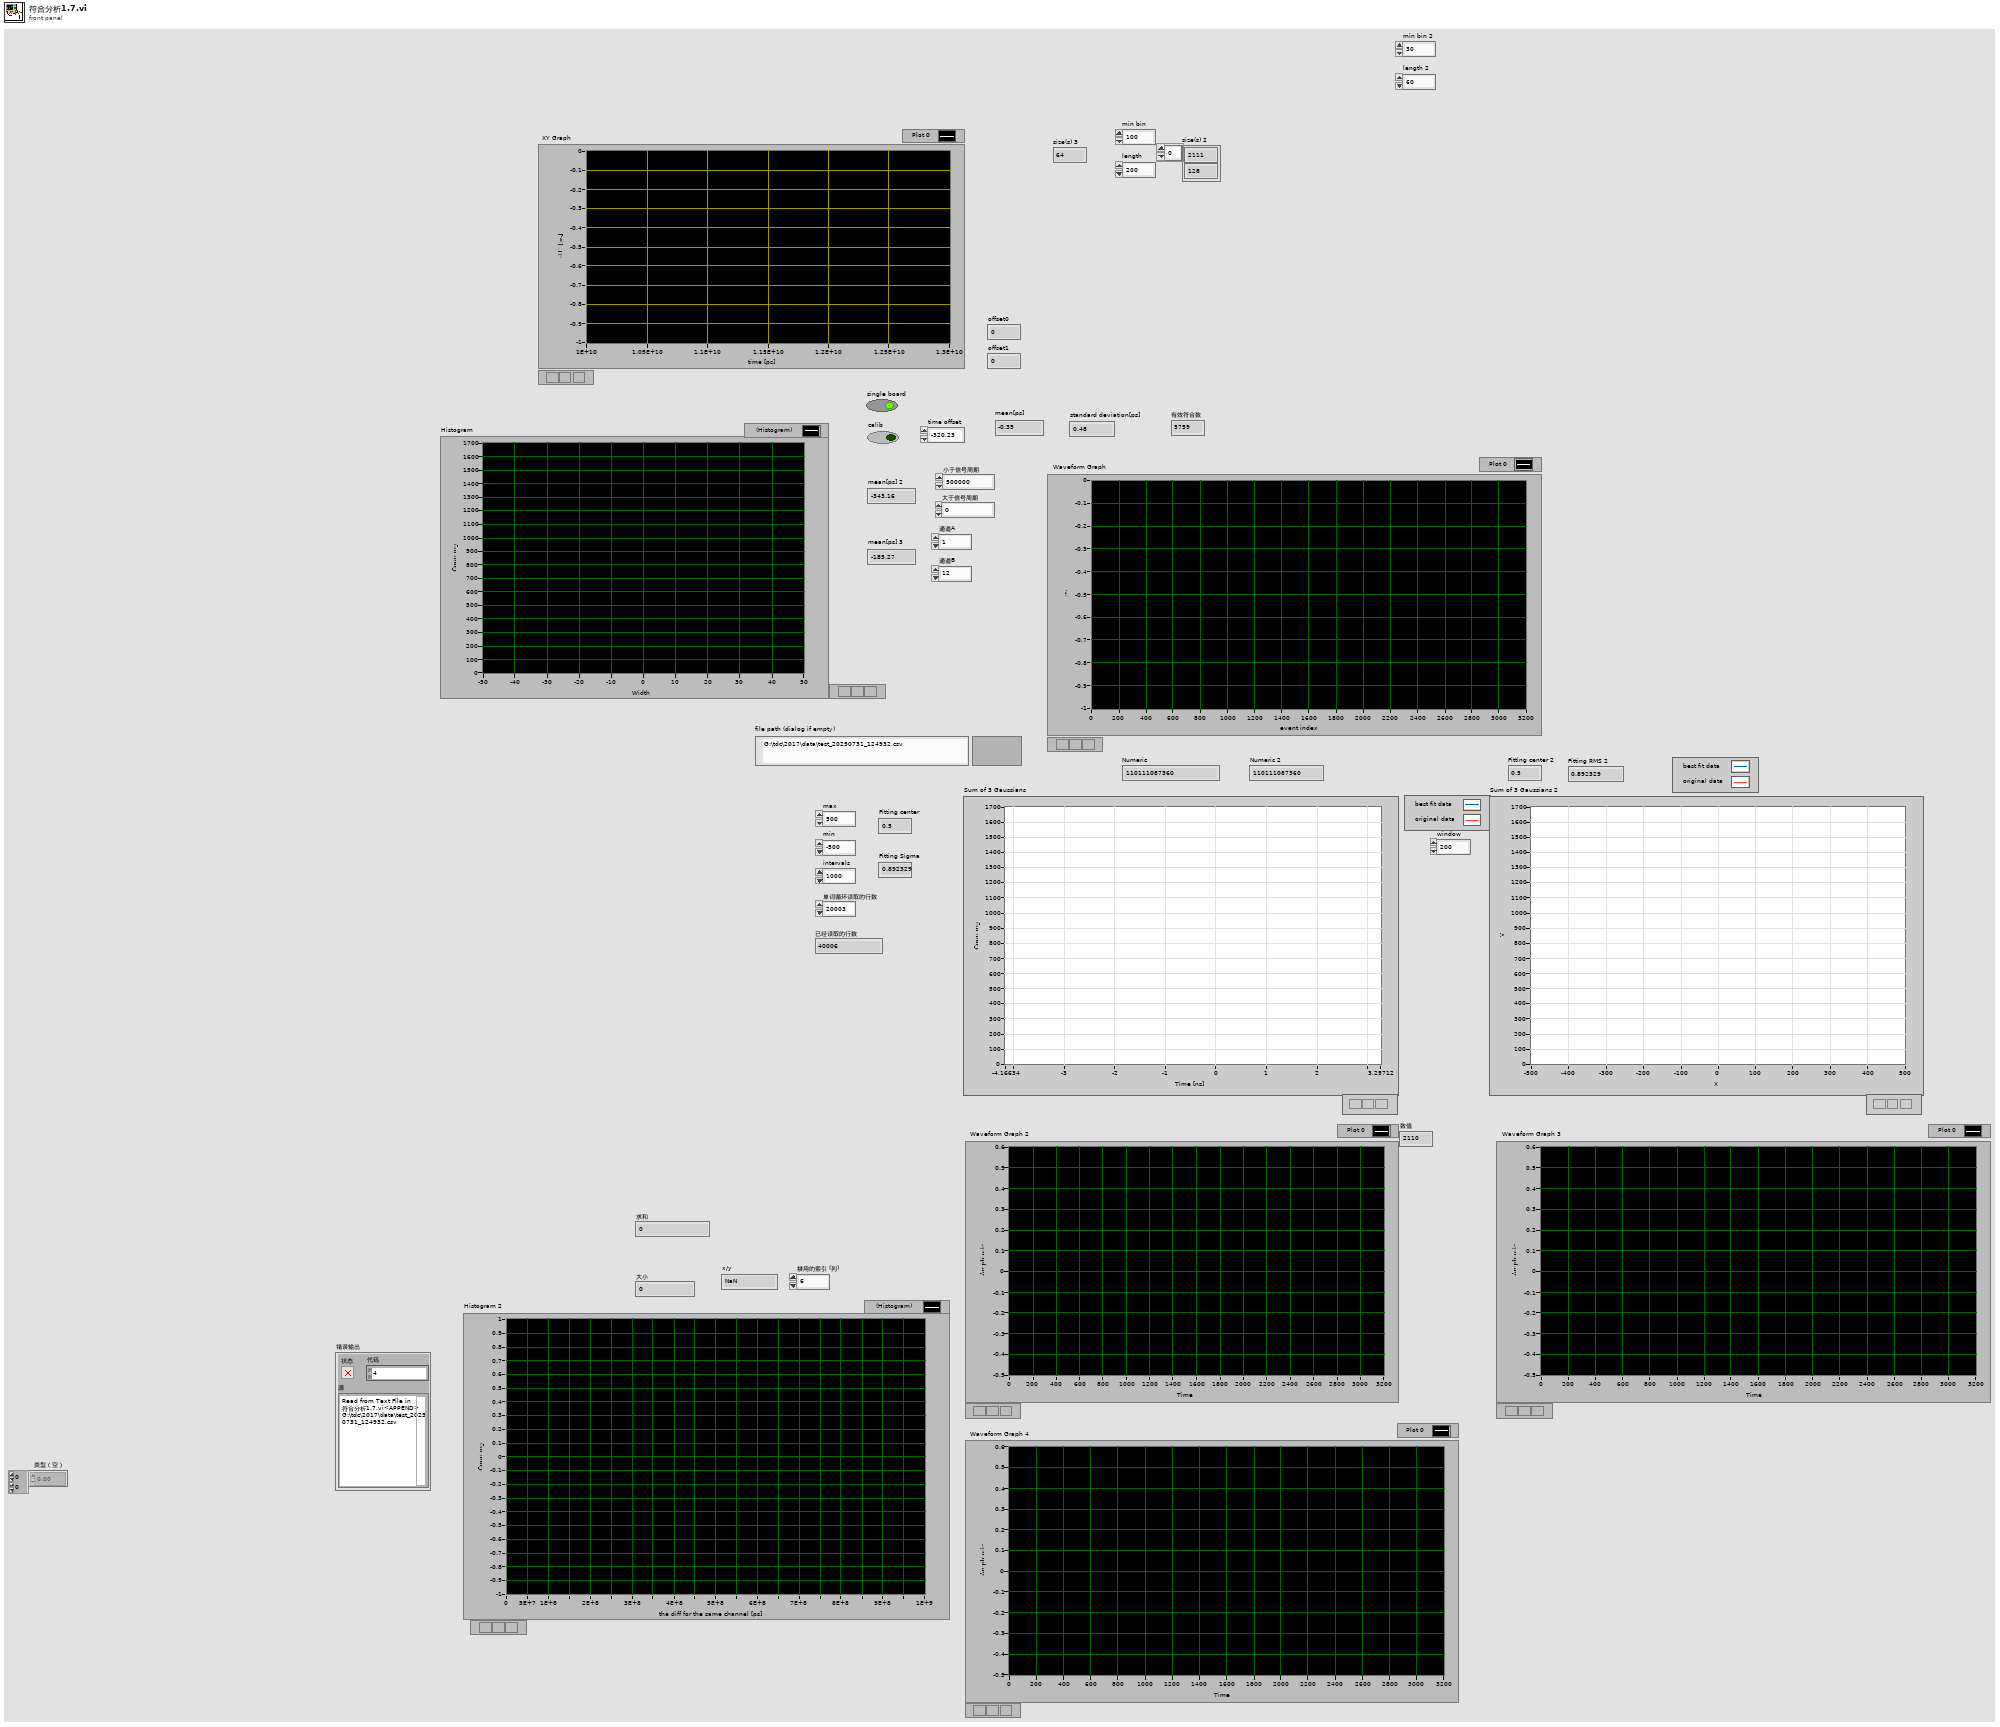
[diagram p1: front panel]
types:
  T1 = cluster{"X Values":dbl[], "Histogram: h(x)":dbl[]}[]
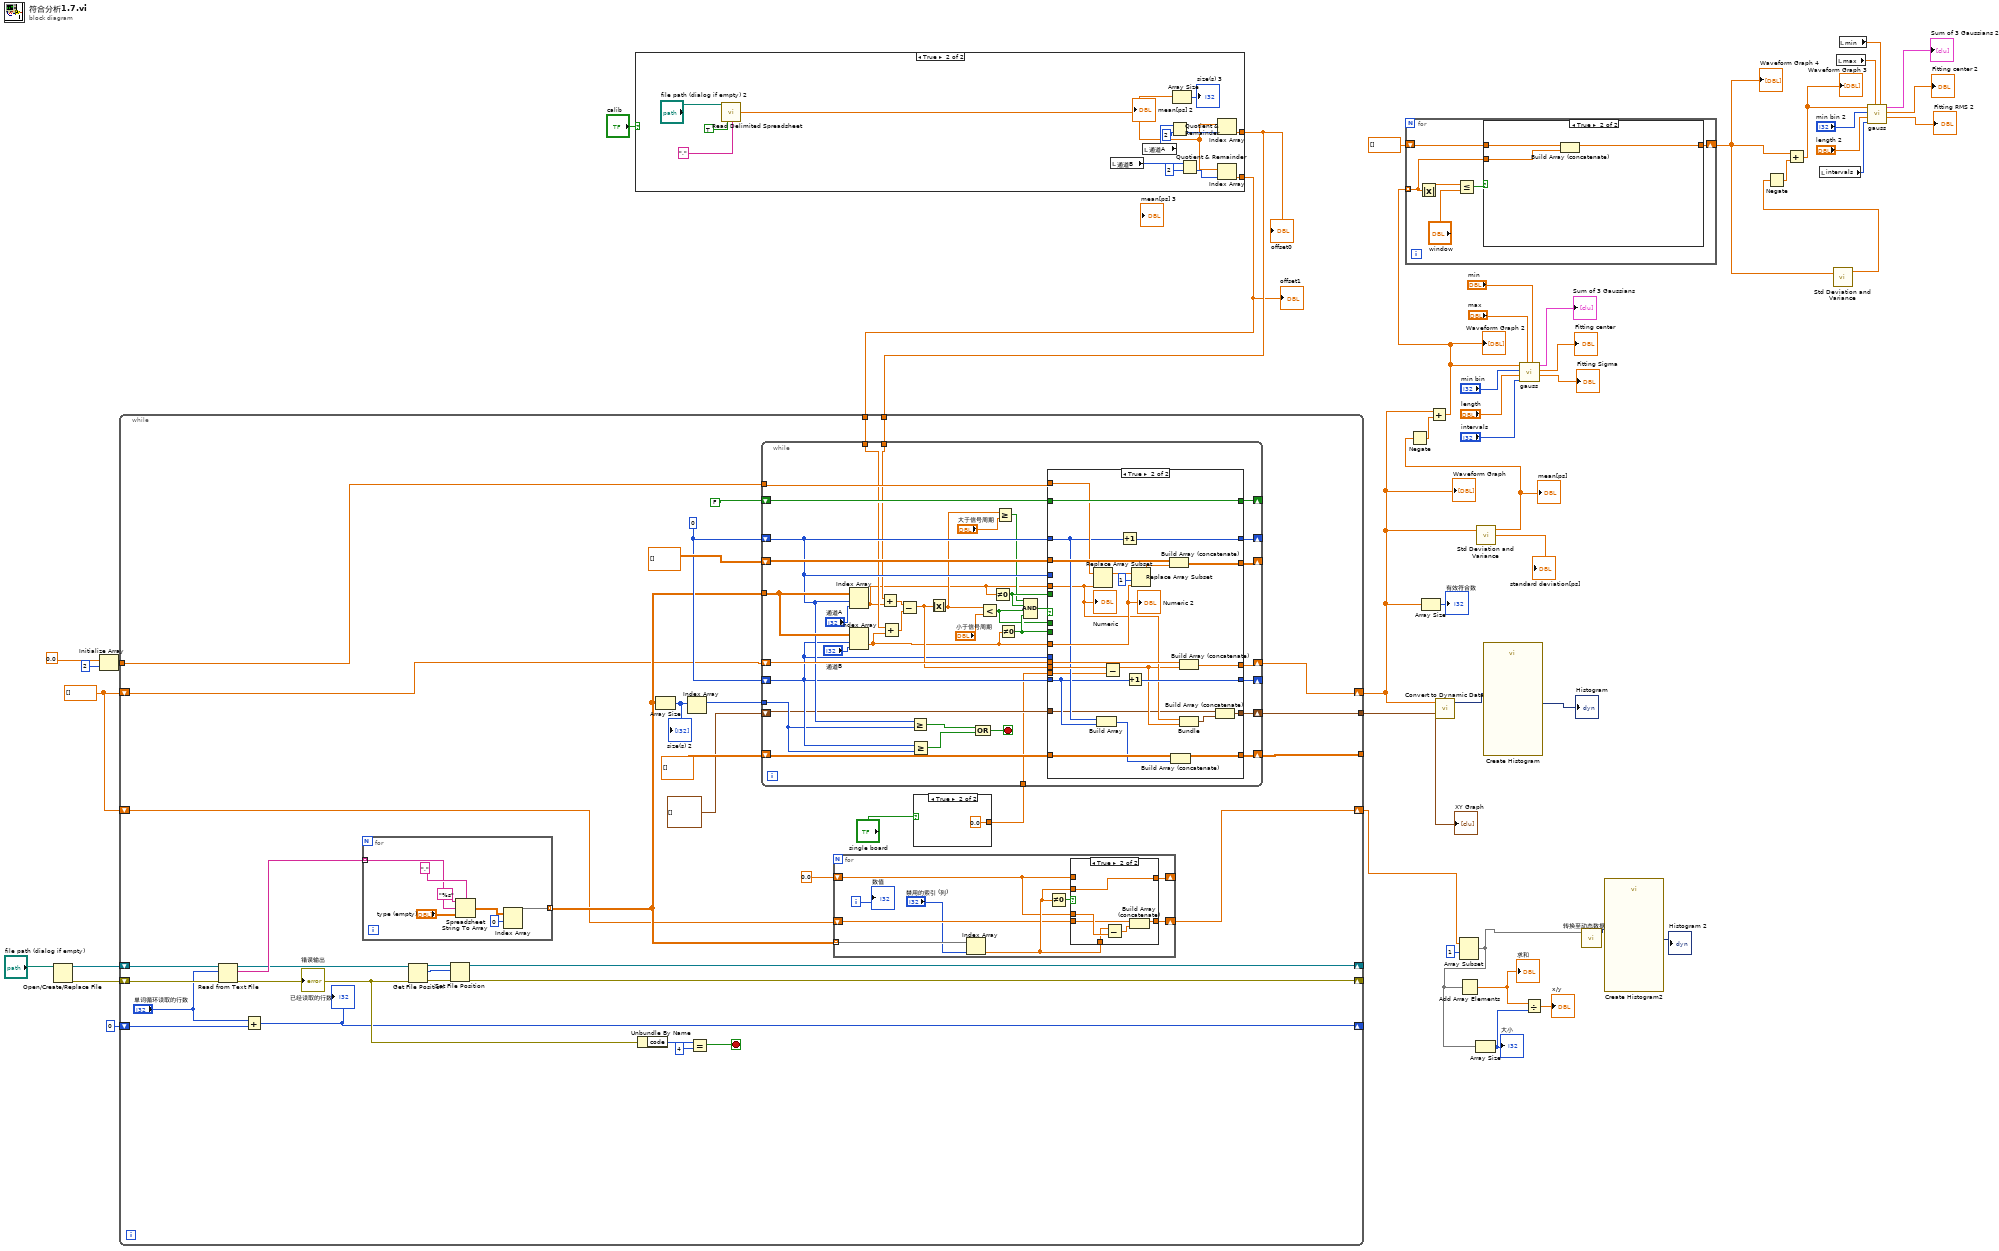
[diagram p0: block diagram]
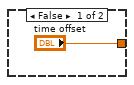
[diagram p2: hidden frame]
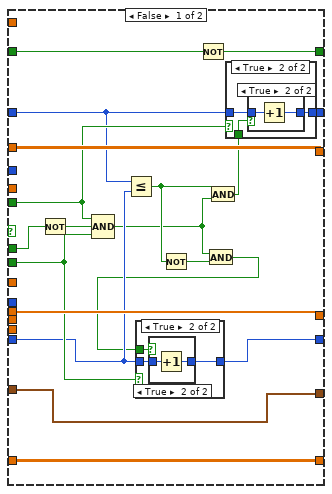
[diagram p4: hidden frame]
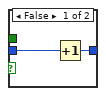
[diagram p5: hidden frame]
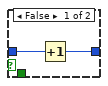
[diagram p7: hidden frame]
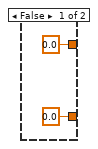
[diagram p9: hidden frame]
diagram:
  w6 = dbl[] []
  n1 = Open/Create/Replace File(file path (use dialog)="file path (dialog if empty)") -> (refnum out=w9:refnum<file>, error out=w8:errorcluster)  [unwired: 5 in, 1 out]
  n2 = Initialize Array(0.0 ("element"), 2 ("dimension size")) -> (w47:dbl[])
  n3 = case shown="True" "calib" {
    tunnel: [0.0 ("Numeric") w62] -> w13
    tunnel: [0.0 ("Numeric") w61] -> w11
    frame False {
    }
    frame True {
      n4 = call-poly <vilib>:"Read Delimited Spreadsheet.vi"("file path (dialog if empty)"="file path (dialog if empty) 2", "transpose? (F)"=TRUE, "delimiter (\\t)"="," ("delimiter (\\t)")) -> ("first row"=w52:dbl[])  [unwired: 7 in, 5 out]
      n5 = local read "通道B"() -> (w57:i32)
      n6 = local read "通道A"() -> (w60:i32)
      n7 = Quotient & Remainder(x=w60, y=2) -> (floor(x/y)=w58:i32)  [unwired: 1 out]
      n8 = Array Size(array=w52) -> (size(s)=→"size(s) 3":i32)
      n9 = Quotient & Remainder(x=w57, y=2) -> (floor(x/y)=w55:i32)  [unwired: 1 out]
      n10 = Index Array(array=w52, index=w58) -> (element=w62:dbl)
      n11 = Index Array(array=w52, index=w55) -> (element=w61:dbl)
    }
  }
  "offset0" <- w13
  "offset1" <- w11
  n12 = while {
    tunnel: [w92] -> w26
    tunnel: [w90] -> _
    tunnel: w13 -> [w88]
    tunnel: w11 -> [w87]
    tunnel: w47 -> [w98]
    shift-right: [w77] -> _
    shift-left: w9 -> [w79]
    shift-right: [w76] -> _
    shift-left: w8 -> [w78]
    shift-right: [w68] -> _
    shift-left: 0 -> [w70]
    shift-right: [w91] -> w22
    shift-left: w6 -> [w67]
    shift-right: [w65] -> w5
    shift-left: w6 -> [w66]
    stop <- w72 stop-if-true
    w95 = 0
    n13 = Read from Text File(file (use dialog)=w79, count="单词循环读取的行数", error in=w78) -> (refnum out=w83:refnum<file>, text=w84:string[], error out=w73:errorcluster)  [unwired: 1 in, 1 out]
    "错误输出" <- w73
    n14 = Add(x="单词循环读取的行数", y=w70) -> (x+y=w68:i32)
    "已经读取的行数" <- w68
    n15 = for {
      tunnel: w84 -> [w104] mode=indexing
      tunnel: [w102] -> w71 mode=indexing
      n16 = Spreadsheet String To Array(delimiter (Tab)="," ("delimiter (\\t)"), format string="%s" ("format (%.3f)"), spreadsheet string=w104, array type (2D Dbl)="type (empty)") -> (array=w103:dbl[][])
      n17 = Index Array(array=w103, index (row)=0 ("索引 (行)")) -> (element=w102:dbl[])  [unwired: 1 in]
    }
    n18 = Get File Position(4:w73, 7:w83) -> (0:w81:errorcluster, 2:w80:i64, 3:w82:refnum<file>)
    n19 = Set File Position(offset (in bytes) (0)=w80, refnum=w82, error in=w81) -> (refnum out=w77:refnum<file>, error out=w76:errorcluster)  [unwired: 1 in]
    n20 = Unbundle By Name(w73) -> ("code"=w75:i32)
    n21 = Array Size(array=w71) -> (size(s)=w97:i32[])
    "size(s) 2" <- w97
    n22 = Index Array(array=w97) -> (element=w96:i32)  [unwired: 1 in]
    n23 = Equal?(x=w75, y=4) -> (x = y?=w72:bool)
    n24 = for {
      tunnel: w71 -> [w118] mode=indexing
      shift-right: [w116] -> _
      shift-left: 0.0 ("Numeric") -> [w111]
      shift-right: [w113] -> w65
      shift-left: w66 -> [w114]
      i -> [w110]
      n25 = Index Array(array=w118, index="禁用的索引 (列)") -> (element=w115:dbl)
      n26 = Not Equal To 0?(x=w115) -> (x != 0?=w117:bool)
      n27 = case shown="True" w117 {
        tunnel: w115 -> [_ w126]
        tunnel: [w120 w126] -> w116
        tunnel: w111 -> [w120 _]
        tunnel: w111 -> [_ w125]
        tunnel: w115 -> [_ w124]
        tunnel: w114 -> [w119 w122]
        tunnel: [w119 w121] -> w113
        frame False {
        }
        frame True {
          n28 = Subtract(x=w124, y=w125) -> (x-y=w123:dbl)
          n29 = Build Array (concatenate)(w122, w123) -> (w121:dbl[])
        }
      }
      "数值" <- w110
    }
    n30 = case shown="True" "single board" {
      tunnel: ["time offset" 0.0 ("time offset")] -> w86
      frame False {
      }
      frame True {
      }
    }
    n31 = while {
      tunnel: w71 -> [w164]
      shift-right: [w160] -> _
      shift-left: w95 -> [w146]
      shift-right: [w157] -> _
      shift-left: w95 -> [w145]
      shift-right: [w158] -> _
      shift-left: FALSE -> [w159]
      shift-right: [w155] -> _
      shift-left: dbl[][] [] -> [w151]
      tunnel: w98 -> [w156]
      tunnel: w96 -> [w142]
      shift-right: [w149] -> w91
      shift-left: w67 -> [w148]
      shift-right: [w140] -> w90
      shift-left: dbl[][] [] -> [w139]
      shift-right: [w138] -> w92
      shift-left: cluster{"Numeric":dbl, dbl}[] [] -> [w137]
      tunnel: w88 -> [w133]
      tunnel: w87 -> [w130]
      tunnel: w86 -> [w127]
      stop <- w152 stop-if-true
      n32 = Index Array(array=w164, index (row)=w146, index (col)="通道A") -> (element=w129:dbl)
      n33 = Index Array(array=w164, index (row)=w145, index (col)="通道B") -> (element=w128:dbl)
      n34 = Add(x=w133, y=w129) -> (x+y=w132:dbl)
      n35 = Add(x=w130, y=w128) -> (x+y=w131:dbl)
      n36 = Subtract(x=w132, y=w131) -> (x-y=w147:dbl)
      n37 = Greater Or Equal?(x=w146, y=w142) -> (x >= y?=w153:bool)
      n38 = Greater Or Equal?(x=w145, y=w142) -> (x >= y?=w154:bool)
      n39 = Absolute Value(x=w147) -> (abs(x)=w136:dbl)
      n40 = Compound Arithmetic op=OR(w153, w154) -> (w152:bool)
      n41 = Less?(x=w136, y="小于信号周期") -> (x < y?=w141:bool)
      n42 = Not Equal To 0?(x=w129) -> (x != 0?=w144:bool)
      n43 = Greater Or Equal?(x=w136, y="大于信号周期") -> (x >= y?=w134:bool)
      n44 = Not Equal To 0?(x=w128) -> (x != 0?=w143:bool)
      n45 = Compound Arithmetic op=AND(w134, w144, w141, w143) -> (w150:bool)
      n46 = case shown="True" w150 {
        tunnel: w146 -> [w170 w208]
        tunnel: [w183 w216] -> w160
        tunnel: w159 -> [w182 w223]
        tunnel: [w181 w223] -> w158
        tunnel: w145 -> [w171 w207]
        tunnel: [w178 w215] -> w157
        tunnel: w151 -> [w180 w222]
        tunnel: w156 -> [_ w221]
        tunnel: w129 -> [_ w205]
        tunnel: w128 -> [_ w211]
        tunnel: [w180 w217] -> w155
        tunnel: [w179 w214] -> w149
        tunnel: w148 -> [w179 w213]
        tunnel: w147 -> [_ w212]
        tunnel: w146 -> [_ _]
        tunnel: w145 -> [_ _]
        tunnel: w144 -> [w177 _]
        tunnel: w143 -> [w176 _]
        tunnel: w141 -> [w175 _]
        tunnel: [w173 w210] -> w140
        tunnel: w139 -> [w173 w209]
        tunnel: [w165 w202] -> w138
        tunnel: w137 -> [w165 w201]
        tunnel: w127 -> [_ w200]
        frame False {
          n47 = Not(x=w175) -> (.not. x?=w174:bool)
          n48 = Compound Arithmetic op=AND(w177, w174, w176) -> (w167:bool)
          n49 = Less Or Equal?(x=w170, y=w171) -> (x <= y?=w168:bool)
          n50 = Not(x=w168) -> (.not. x?=w169:bool)
          n51 = Not(x=w182) -> (.not. x?=w181:bool)
          n52 = And(x=w167, y=w169) -> (x .and. y?=w166:bool)
          n53 = case shown="True" w176 {
            tunnel: w171 -> [w185 w188]
            tunnel: [w184 w187] -> w178
            tunnel: w166 -> [_ w186]
            frame False {
              n54 = Increment(x=w185) -> (x+1=w184:i32)
            }
            frame True {
              n55 = case shown="True" w186 {
                tunnel: w188 -> [w189 w191]
                tunnel: [w189 w190] -> w187
                frame False {
                }
                frame True {
                  n56 = Increment(x=w191) -> (x+1=w190:i32)
                }
              }
            }
          }
          n57 = And(x=w168, y=w167) -> (x .and. y?=w172:bool)
          n58 = case shown="True" w177 {
            tunnel: w170 -> [w193 w196]
            tunnel: [w192 w195] -> w183
            tunnel: w172 -> [_ w194]
            frame False {
              n59 = Increment(x=w193) -> (x+1=w192:i32)
            }
            frame True {
              n60 = case shown="True" w194 {
                tunnel: w196 -> [w197 w199]
                tunnel: [w197 w198] -> w195
                frame False {
                }
                frame True {
                  n61 = Increment(x=w199) -> (x+1=w198:i32)
                }
              }
            }
          }
        }
        frame True {
          n62 = Replace Array Subset(array=w221, new element=w205) -> (w220:dbl[])  [unwired: 1 in]
          n63 = Build Array(w208, w207) -> (w206:i32[])
          n64 = Subtract(x=w212, y=w200) -> (x-y=w204:dbl)
          n65 = Increment(x=w208) -> (x+1=w216:i32)
          n66 = Increment(x=w207) -> (x+1=w215:i32)
          n67 = Replace Array Subset(array=w220, new element=w211, index=1) -> (w218:dbl[])
          n68 = Build Array (concatenate)(w222, w218) -> (w217:dbl[][])
          n69 = Build Array (concatenate)(w209, w206) -> (w210:dbl[][])
          n70 = Build Array (concatenate)(w213, w204) -> (w214:dbl[])
          n71 = Bundle(w205, w204) -> (w203:cluster{dbl, dbl})  [unwired: 1 in]
          n72 = Build Array (concatenate)(w201, w203) -> (w202:cluster{"Numeric":dbl, dbl}[])
          "Numeric" <- w205
          "Numeric 2" <- w211
        }
      }
    }
  }
  "Waveform Graph" <- w22
  "XY Graph" <- w26
  n73 = Array Size(array=w22) -> (size(s)=→"有效符合数":i32)
  n74 = call "Convert to Dynamic Data"("Array"=w22) -> ("Dynamic Data Type"=w45:dynamicdata)  [unwired: 3 in]
  n75 = Array Subset(array=w5, index=1) -> (w1:dbl[])  [unwired: 1 in]
  n76 = Add Array Elements(numeric array=w1) -> (sum=w3:dbl)
  "求和" <- w3
  n77 = Array Size(array=w1) -> (size(s)=w4:i32)
  "大小" <- w4
  n78 = call <vilib>:"Std Deviation and Variance.vi"("X"=w22) -> ("mean"=w37:dbl, "standard deviation"=→"standard deviation[ps]":dbl)  [unwired: 1 in, 1 out]
  "mean[ps]" <- w37
  n79 = Negate(x=w37) -> (-x=w14:dbl)
  n80 = Add(x=w22, y=w14) -> (x+y=w21:dbl[])
  "Waveform Graph 2" <- w21
  n81 = for {
    tunnel: w21 -> [w228] mode=indexing
    shift-right: [w226] -> w27
    shift-left: dbl[] [] -> [w227]
    n82 = Absolute Value(x=w228) -> (abs(x)=w224:dbl)
    n83 = Less Or Equal?(x=w224, y="window") -> (x <= y?=w229:bool)
    n84 = case shown="True" w229 {
      tunnel: w228 -> [_ w232]
      tunnel: w227 -> [w230 w233]
      tunnel: [w230 w231] -> w226
      frame False {
      }
      frame True {
        n85 = Build Array (concatenate)(w233, w232) -> (w231:dbl[])
      }
    }
  }
  "Waveform Graph 4" <- w27
  n86 = call "Create Histogram"("Signal"=w45) -> ("Histogram"=→"Histogram":dynamicdata)  [unwired: 9 in, 1 out]
  n87 = call "gauss.vi"("min"="min", "max"="max", "intervals"="intervals", "length"="length", "low"="min bin", "Waveform Graph"=w21) -> ("standard deviation"=→"Fitting Sigma":dbl, "center"=→"Fitting center":dbl, "Sum of 3 Gaussians"=→"Sum of 3 Gaussians":T1)  [unwired: 3 in]
  n88 = Divide(x=w3, y=w4) -> (x/y=→"x/y":dbl)
  n89 = call "转换至动态数据"("Array"=w1) -> ("Dynamic Data Type"=w17:dynamicdata)  [unwired: 3 in]
  n90 = call "Create Histogram2"("Signal"=w17) -> ("Histogram"=→"Histogram 2":dynamicdata)  [unwired: 9 in, 1 out]
  n91 = local read "intervals"() -> (w18:i32)
  n92 = call <vilib>:"Std Deviation and Variance.vi"("X"=w27) -> ("mean"=w28:dbl)  [unwired: 1 in, 2 out]
  n93 = Negate(x=w28) -> (-x=w34:dbl)
  n94 = Add(x=w27, y=w34) -> (x+y=w35:dbl[])
  "Waveform Graph 3" <- w35
  n95 = local read "max"() -> (w19:dbl)
  n96 = local read "min"() -> (w20:dbl)
  n97 = call "gauss.vi"("min"=w20, "max"=w19, "intervals"=w18, "length"="length 2", "low"="min bin 2", "Waveform Graph"=w35) -> ("standard deviation"=→"Fitting RMS 2":dbl, "center"=→"Fitting center 2":dbl, "Sum of 3 Gaussians"=→"Sum of 3 Gaussians 2":T1)  [unwired: 3 in]
